vi "AlliGator Files Actions.vi"(0 "AlliGator Q Elements in":T7[](array[typedef]), 1 "VI in":refnum<vi>, 2 "Script in":bool, 5 "AlliGator IV DVR":refnum<data-value>, 7 "AlliGator Q Event in":T8=enum."GUI:Idle", 9 "Data":variant, 11 "error in (no error)":errorcluster, 12 "AlliGator Ctrl Refnums":T9) -> (3 "Script out":bool, 4 "AlliGator Q Elements out":T7[](array[typedef]), 6 "AlliGator IV DVR":refnum<data-value>, 10 "[Notebook Message]":T2[](array[typedef]) {"Message Style"."Font Size" min=6.0 step=1.0}, 15 "error out":errorcluster)   [LabVIEW 2021, in "AlliGator Action Engine.lvlib"]
doc: "Processes AlliGator files-related actions."
uses:
  AlliGator Action Engine.lvlib
  AlliGator Q Event.ctl
  GUI/AlliGator Ctrl Refnums.ctl
  GUI/AlliGator Other Ctrl Refnums.ctl
  GUI/AlliGator State Indicator.ctl
  GUI/AlliGator Main Window Tabs.ctl
  GUI/AlliGator Phasor Plot Ctrl Refnums.ctl
  GUI/AlliGator Phasor Graph Ctrl Refnums.ctl
  Phasor/Phasor Calibration Type.ctl
  GUI/AlliGator Dataset Ctrl Refnums.ctl
  Source Image/AlliGator Displayed Image.ctl
  GUI/AlliGator Registered Events Ctrl Refnums.ctl
  GUI/AlliGator Image Histogram Control Refnums.ctl
  Histograms/Linear Histogram Options.ctl
  Histograms/Histogram Bin Option.ctl
  Histograms/Histogram Bin Position.ctl
  Decay Fit Parameter Map/AlliGator Decay Fit Map Control Refnums.ctl
  Fits/IRF(X)PSED/Decay Fit Parameters & Derived Quantities List v2.ctl
  Parameter Map/AlliGator Parameter Map Control Refnums.ctl
  AlliGator Q Element.ctl
  Internal Variables/AlliGator Internal Variables v2.ctl
  <vilib>/vision/Image Controls.llb/IMAQ Image.ctl
  Internal Variables/AlliGator Gate Image Set.ctl
  Files/AlliGator FLI Dataset Type.ctl
  Files/AlliGator Data Series Type.ctl
  Dual-Channel Datasets/AlliGator Dataset Channel.ctl
  Settings/AlliGator Gate Arithmetic.ctl
  Image/Named ROI Description.ctl
  Phasor Graph/AlliGator Decay Metadata v3.ctl
  Decay Analysis/Decay Preprocessing/AlliGator Decay Background Subtraction Info.ctl
  Decay Analysis/Decay Preprocessing/AlliGator Baseline Subtraction Method.ctl
  Graphs/XY Graph/XY Graph Plot Shift Parameters.ctl
  Graphs/XY Graph/XY Graph Plot Shift Method.ctl
  Decay Analysis/Decay Preprocessing/AlliGator Decay Extrapolation Parameters.ctl
  Phasor/Calibration Phasor (m, phi).ctl
  Phasor/Phasor Reference Series.ctl
  Phasor/Phasor Calibration Map v2.ctl
  Phasor/Phasor (g, s).ctl
  Phasor Graph/AlliGator Raw Phasor Plot Data v5.ctl
  Phasor/Phasor Standard Deviation Options.ctl
  Phasor Plot/AlliGator Phasor Multi-Harmonic Data.ctl
  Phasor/Phasor Harmonic Data.ctl
  Decay Fit Parameter Map/AlliGator Decay Fit Options & Parameters v4.ctl
  Fits/IRF(X)PSED/Decay Fit Options v4.ctl
  Fits/Decay Convolution/Decay Model.ctl
  Fits/Residual Type.ctl
  Fits/IRF(X)PSED/Fit Weights Type v2.ctl
  Fits/Non-linear Fitting Method v2.ctl
  Fits/Fit Calculation Method.ctl
  Fits/Non-linear Fitting Algorithm.ctl
  Decay Analysis/Decay Fit/AlliGator Decay Fit Parameter Constraints 2.ctl
  Fits/IRF(X)PSED/Decay Fit Parameters In List.ctl
  Fits/IRF(X)PSED/MLE Baseline Offset Type.ctl
  Decay Analysis/Decay Preprocessing/AlliGator Decay Preprocessing Parameters.ctl
  Fits/IRF(X)PSED/Decay Fit Result Constraint.ctl
  Decay Fit Parameter Map/AlliGator Parameter Maps Data.ctl
  Notebook/Notebook Message Object.ctl
  Rich Text Box/Text Formatting.ctl
  Rich Text Box/Text Colors.ctl
  Rich Text Box/Text Style.ctl
  Rich Text Box/Text Alignment.ctl
  Rich Text Box/Text Format List.ctl
  GUI/AlliGator Windows List.ctl
  Alligator Elements Order in Action Stack.ctl
  Files/AlliGator Export Dataset Options.ctl
  Globals, Variables, Constants/AlliGator Variables List.ctl
  Files/AlliGator Load Dataset Options.ctl
  Files/AlliGator Single Image File Info.ctl
  Source Image/AlliGator Image Type.ctl
  Files/AlliGator Folder Selection.ctl
  Files/AlliGator Select Folder Mode.ctl
  Scripts/AlliGator Data Load & Process Options.ctl
  Scripts/AlliGator Data Information.ctl
  Settings/AlliGator Background Subtraction Parameters.ctl
  Settings/AlliGator Define Gates to.ctl
  Settings/AlliGator Gates to Keep.ctl
  Scripts/AlliGator Source Image Settings.ctl
  Settings/AlliGator Low Count Pixels Rejection Options.ctl
  Settings/AlliGator High Count Pixels Rejection Options.ctl
  Settings/AlliGator Image Smoothing Options.ctl
  Arrays/Kernel Type.ctl
  Arrays/Smoothing Algorithm.ctl
  Source Image/AlliGator Image Binning Options.ctl
  Decay Analysis/Decay Preprocessing/AlliGator Decay Preprocessing Options.ctl
  Decay Analysis/Decay Preprocessing/AlliGator Background Subtraction Parameters.ctl
  Settings/AlliGator Settings List.ctl
  Globals, Variables, Constants/AlliGator Globals.vi
  AlliGator Add Action Array to Stack.vi
  Variant/Variant to Data/Variant to I32.vi
  Variant/Variant to Data/Variant to Path.vi
  AlliGator Add Single Action to Stack.vi
  Variant/Variant to Data/Variant to DBL.vi
  Variant/Variant to Data/Variant to Data.lvlib
  GUI/AlliGator GUI.lvlib
  Utilities/Utilities.lvlib
  GUI/GUI.lvlib
  Files/AlliGator Files.lvlib
  Source Image/AlliGator Source Image.lvlib
  Scripts/AlliGator Scripts.lvlib
  Graphs/XY Graph/XY Graph Add-Ons.lvlib
  Decay Analysis/Decay Preprocessing/AlliGator Decay Preprocessing.lvlib
  Arrays/Arrays.lvlib
  Settings/AlliGator Settings.lvlib
  Globals, Variables, Constants/AlliGator Globals, Variables & Constants.lvlib
  Image/Image.lvlib
  Notebook/Notebook.lvlib
  Phasor/Phasor.lvlib
  Decay Fit Parameter Map/AlliGator Decay Fit Parameter Map.lvlib
  Phasor Graph/AlliGator Phasor Graph.lvlib
  Internal Variables/AlliGator Internal Variables.lvlib
  Phasor Plot/AlliGator Phasor Plot.lvlib
  Fits/Fits.lvlib
  Decay Analysis/Decay Fit/AlliGator Decay Fit.lvlib
  Rich Text Box/Rich Text Box.lvlib
  Dual-Channel Datasets/AlliGator Dual-Channel Datasets.lvlib
  Histograms/Histogram Window.lvlib
  Parameter Map/AlliGator Parameter Map.lvlib
panel:
  in  "Displayed Image 2":T1=enum."Sum of All Gates" caption="Displayed Image"
  in  "Displayed Image":T1=enum."Sum of All Gates"
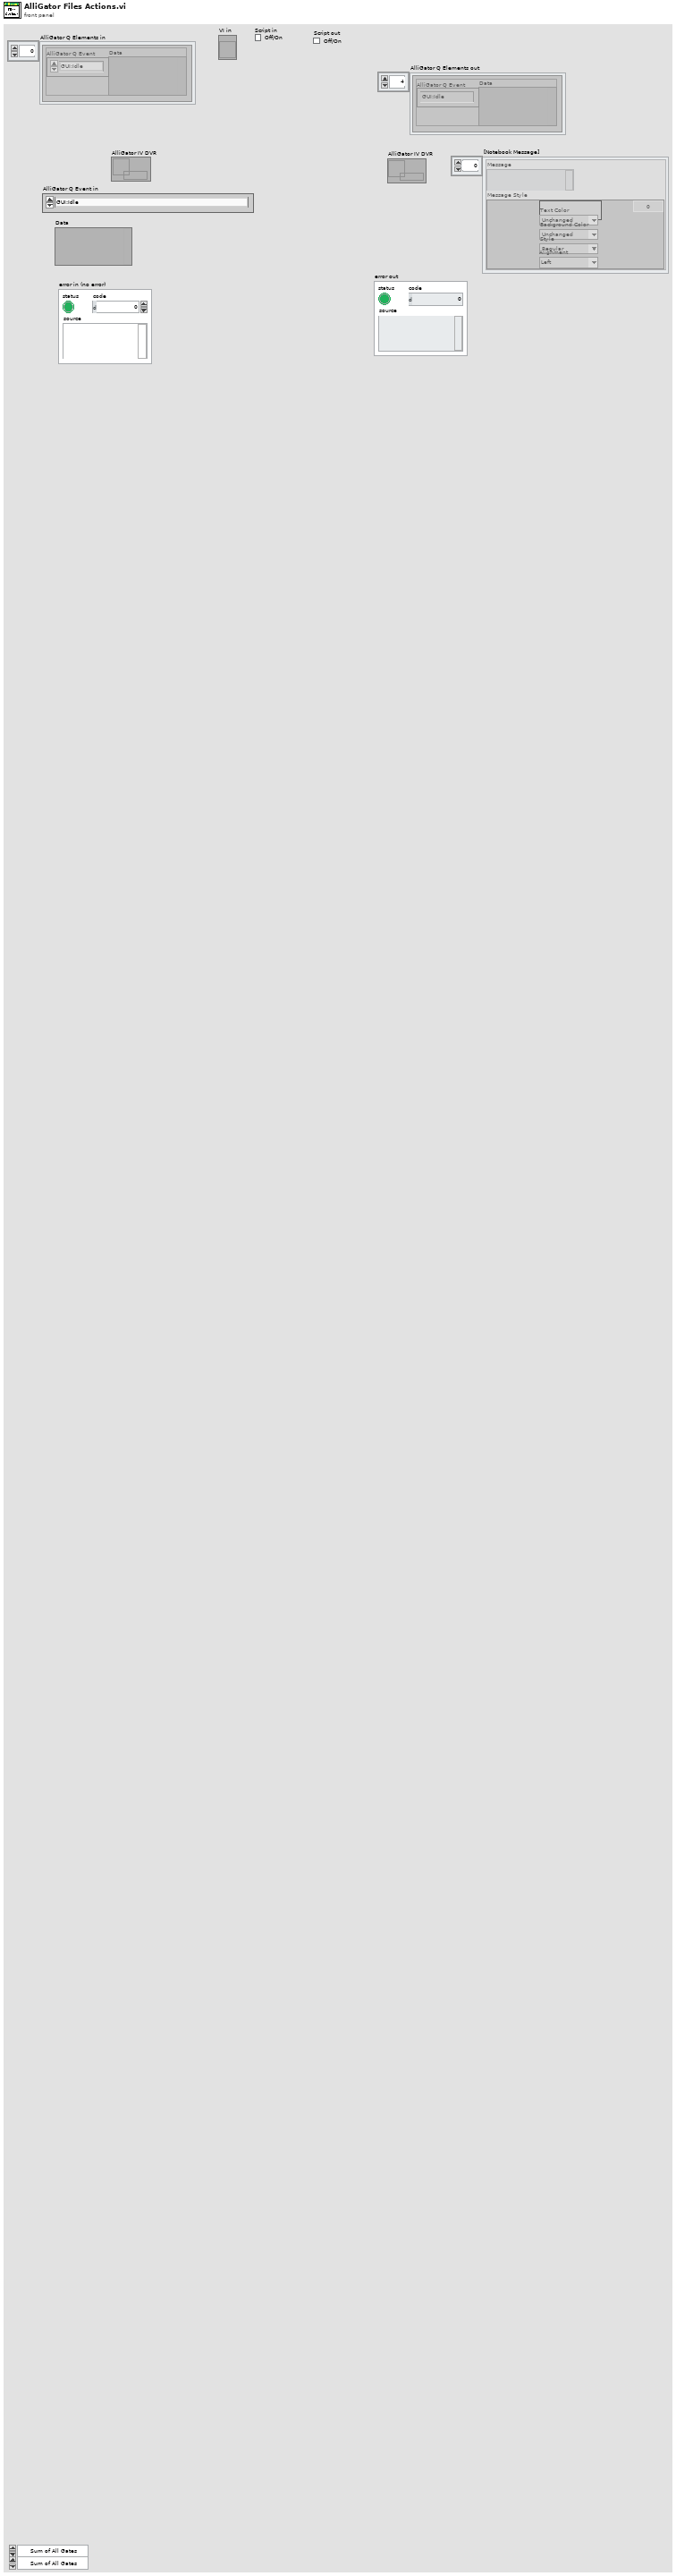
[diagram p1: front panel]
types:
  T1 = typedef "AlliGator Source Image.lvlib/AlliGator Displayed Image.ctl" = enum16{"Single Gate", "Sum of All Gates", "Max of All Gates", "Min of All Gates", "-", "White Ligth Image", "Mask Image"}
  T2 = typedef "Notebook.lvlib/Notebook Message Object.ctl" = cluster{"Message":string, "Message Style":T3}
  T3 = typedef "Rich Text Box.lvlib/Text Formatting.ctl" = cluster{"Font":string, "Text Color":T4, "Background Color":T4, "Style":T5, "Font Size":dbl, "Alignment":T6}
  T4 = typedef "Rich Text Box.lvlib/Text Colors.ctl" = enum16{"Unchanged", "Black", "Blue", "Cyan", "Maroon", "Gray", "Violet", "Green", "Light Green", "Orange", "Yellow", "Magenta", "Red", "White"}
  T5 = typedef "Rich Text Box.lvlib/Text Style.ctl" = enum16{"Regular", "Bold", "Italic", "Underline", "Strikeout"}
  T6 = typedef "Rich Text Box.lvlib/Text Alignment.ctl" = enum16{"Left", "Right", "Center"}
  T7 = typedef "AlliGator Action Engine.lvlib/AlliGator Q Element.ctl" = cluster{"AlliGator Q Event":T8, "Data":variant}
  T8 = typedef "AlliGator Action Engine.lvlib/AlliGator Q Event.ctl" = enum16{"---- Files ----", "Files:Set Batch Export Files To Save", "Files:Set Dataset Loading & Pre-processing Options", "Files:Check #Frames in Dataset", "Files:Increment Frame Index", "Files:Open Mask Image", "Files:Open White Light Image", "Files:Open Single Dataset", "Files:New Folder of Folders Selected", "Files:Load File (all Types)_Scriptable", "Files:Move Flattened Series to Folders Series", "Files:Select Folder", "Files:Load FLI Dataset", "Files:Load Swiss SPAD 1 Dataset", "Files:Load Swiss SPAD 2 Dataset", "Files:Load .sdt FLI Dataset", "Files:Load .ptu FLI Dataset", "Files:Load .bin FLI Dataset", "Files:Load Single Gate Image Folder", "Files:Load I/m/phi Dataset (deprecated)", "Files:Load Single Image", "Files:Subtract Background File", "Files:Export FLI Dataset", "Files:Load HDF5 FLI Dataset", "Files:Set Destination File Path", "Files:Save Mask Image", "Files:Batch Conversion", "Files:New Folder Selected", "Files:Close FLI Dataset", "Files:Close FLI Dataset Series", "Files:Close White Light Image", "Files:Close Mask Image", "---- FLI Dataset ----", "FLI Dataset:Channel Arithmetic", "FLI Dataset:Export Average Lifetime Map as ASCII", "FLI Dataset:Export User-Defined Quantity Map as ASCII", "FLI Dataset:Python Function FLI Dataset Event", "FLI Dataset:ROI Analysis", "FLI Dataset:Tilted Logistic Square Gated IRF Characteristics Map", "FLI Dataset:Logistic Square Gated IRF Characteristics Map", "FLI Dataset:Square Gated IRF Characteristics Map", "FLI Dataset:Multi-ROI Single-Pixel Phasor Analysis", "FLI Dataset:Multi-ROI Single-Pixel NLSF Analysis", "FLI Dataset:All ROIs IRF Extraction", "FLI Dataset:All ROIs Decay Fit Non-Interactive (Fast + Individual IRF)", "FLI Dataset:All ROIs Phasor Analysis", "FLI Dataset:All ROIs Decay Fit", "FLI Dataset:Fluorescence Decay Statistics", "FLI Dataset:Update Decay Statistics Graph", "FLI Dataset:Get Decay from ROI", "FLI Dataset:All ROIs Average Lifetimes", "FLI Dataset:Save/Load Local IRFs", "FLI Dataset:Clear Local IRFs", "FLI Dataset:Phasor Calibration Maps (# Gates Series) Script", "FLI Dataset:Calibrated Phasor Map Series", "---- FLI Dataset Series ----", "FLI Dataset Series:Sum All Datasets in Series", "FLI Dataset Series:Add Dataset to Accumulated Dataset", "FLI Dataset Series:Display Accumulated Dataset", "FLI Dataset Series:Clear Dataset Series Sum", "FLI Dataset Series:Time-Series Analysis (NLSF)", "FLI Dataset Series:Time-Series Analysis (Phasor)", "---- Image ----", "Image:Update Image Profile Plots", "Image:Image Histogram Cursor Move", "Image:Image Histogram", "Image:Image Contrast", "Image:Set Image Histogram Cursor Move Flag", "Image:Clear Image Overlay", "Image:Use ROI as Search Area", "Image:Set ROI Diameter", "Image:Save Image Data as TIFF", "Image:Save Displayed Image with Overlay", "Image:Save Image Overlay Only", "Image:Save Image as Hot Pixel Mask", "Image:Change Source Image Color Palette", "Image:Copy Image to Clipboard", "Image:Source Image ROI Selection", "Image:Delete All ROIs", "Image:Delete All Unselected ROIs", "Image:Delete ROI", "Image:Merge All ROIs", "Image:Store ROI", "Image:Source Image ROI Storage", "Image:Export ROI Description to Notebook", "Image:Save ROI", "Image:Load ROI", "Image:Paste ROI Definition", "Image:Clear ROI", "Image:Identify ROIs in Mask Image", "Image:Create Complementary ROI", "Image:Create Contour ROI", "Image:Create ROI(s) from Pixels with Peak above Min_Scriptable", "Image:Create ROI(s) from Pixels with Intensity above Min_Scriptable", "Image:Compute ROI Statistics", "Image:Delete ROI(s) based on ROI Characteristics", "Image:Create ROI Grid", "Image:ROI to Individual Pixel ROIs", "Image:Python Function Source Image Event", "Image:Show Phasor Calibration Map ROI Centers", "Image:Convert ROI to Mask Image", "Image:Mouse Move", "Image:Mouse Up", "Image:Set Source Image Mouse Move Flag", "Image:Add Scale Bar Overlay", "Image:Delete Existing ROIs Option", "Image:Overlay ROI Median", "Image:Check Current ROI", "Image:Update True Pixel Value", "---- Decay ----", "Decay:Clear IRF/Reference Plot", "Decay:Add Decay to Graph", "Decay:Smoothen Plot", "Decay:Smoothen Plot Tail", "Decay:Average Selected Plots", "Decay:Extract IRF", "Decay:Optimal IRF Extraction", "Decay:Threshold IRF", "Decay:Fit to Model IRF", "Decay:Fit IRF to Square Gate", "Decay:Fit IRF to Logistic Square Gate", "Decay:Fit IRF to Tilted Logistic Square Gate", "Decay:Create Bounding Cursors Set", "Decay:Export Bounding Cursors Definition to Notebook", "Decay:Denoise Plot", "Decay:Compute Cumulative Function", "Decay:Use as Reference Decay", "Decay:Show Reference Decay/IRF", "Decay:Extrapolate Decay", "Decay:Create Head & Tail Bounding Cursors", "Decay:Store Cursor-defined Head & Tail Fractions", "Decay:Rebin Plot", "Decay:1-Normalize Decay", "Decay:[0-1]-Normalize Plot", "Decay:Straighten Decay", "Decay:Shift Decay", "Decay:Fold Decay", "Decay:Fit Decay", "Decay:Global Fit of Selected Decays", "Decay:Post Global Fit Script", "Decay:Add Global Fit Parameters to Graph", "Decay:Add Decay Parameter(s) to Plot (Graph)", "Decay:Export Decay to Phasor Graph", "Decay:Compute Average Lifetime", "Decay:Plot Convolution", "Decay:Graph Tip Strip Update", "---- Decay Statistics ----", "Decay Statistics:Tip Strip Update", "---- Intensity Time Trace ----", "Intensity Time Trace:Use File Timestamp", "Intensity Time Trace:Load Intensity Corrections File", "Intensity Time Trace:Clear Intensity Corrections File", "Intensity Time Trace:Tip Strip Update", "---- Phasor Plot ----", "Phasor Plot:Build Phasor Plot", "Phasor Plot:Change Phasor Plot Color Palette", "Phasor Plot:Adjust Phasor Plot Display Range", "Phasor Plot:Highlight Image ROI in Phasor Plot", "Phasor Plot:Save Phasor Plot Image with Overlay", "Phasor Plot:Export Complex Phasor Map", "Phasor Plot:Export Phasor Ratio Map", "Phasor Plot:Export Average Lifetime Map", "Phasor Plot:Compute Phase Lifetime Histogram", "Phasor Plot:Compute Phasor Ratio Histogram", "Phasor Plot:Compute Phase Lifetime vs Intensity Scatter Plot", "Phasor Plot:Weber 2-Component Decomposition", "Phasor Plot:Update Phasor Color Map Vertices", "Phasor Plot:Clear Phasor Overlay", "Phasor Plot:Use Segment Extremities as References", "Phasor Plot:Use UC/Segment Intersections as References", "Phasor Plot:Use UC/Principal Axis Intersections as References", "Phasor Plot:Use UC/Linear Fit Intersections as References", "Phasor Plot:Update Phasor Plot Reference", "Phasor Plot:Show Local Phasor Info in Phasor Plot", "Phasor Plot:Update Phasor Plot State", "Phasor Plot:Phasor Plot ROI Storage", "Phasor Plot:Phasor Plot ROI Selection", "Phasor Plot:Python Function Phasor Plot Event", "Phasor Plot:Overlay Phasor ROI, Ratio or Map in Source Image", "Phasor Plot:Compute Decay of Selected Phasors", "Phasor Plot:Phasor at Image Pixel", "Phasor Plot:Mouse Move", "Phasor Plot:Mouse Up", "Phasor Plot:Display Range Mouse Move", "Phasor Plot:Set Mouse Move Flag", "Phasor Plot:Update True Phasor Plot Value", "---- Phasor Graph ----", "Phasor Graph:Get Phasor Value", "Phasor Graph:Create New Phasor Plot Dialog", "Phasor Graph:Update Last Phasor Value", "Phasor Graph:Update Phasor (m, phi)", "Phasor Graph:Remove Single Phasor from Plot", "Phasor Graph:Add Single Phasor to Plot", "Phasor Graph:Remove Phasor Plot", "Phasor Graph:Remove Selected Phasor Plots", "Phasor Graph:Clear Phasor Data", "Phasor Graph:Clear Phasor Graph", "Phasor Graph:Cursor Move", "Phasor Graph:Draw Cursor Connecting Line", "Phasor Graph:Clear Cursor Connecting Line", "Phasor Graph:Find UC Intersection", "Phasor Graph:Use UC/Cursor-Defined Line Intersections", "Phasor Graph:Use Selected Plots Fitted Line/UC Intersections", "Phasor Graph:Use Selected Plots Principal Axis/UC Intersections", "Phasor Graph:Show Single Phasor", "Phasor Graph:Save Single Phasor Plot", "Phasor Graph:Save All Phasor Plots", "Phasor Graph:Load Phasor Plot(s)", "Phasor Graph:Phasor Multiplication", "Phasor Graph:Compute Average Phasor", "Phasor Graph:Compute Multiple Average Phasors (Selected Plots)", "Phasor Graph:Export Single Phasor Plot Phase Lifetimes", "Phasor Graph:Parameter 2 vs Parameter 1 Scatter Plot", "Phasor Graph:Use Cursor n Location", "Phasor Graph:Set Reference n to Current Phase Lifetime Value", "Phasor Graph:Set Reference n to Lifetime Value", "Phasor Graph:Set Cursor n Location", "Phasor Graph:Save Phasor Graph Image", "Phasor Graph:Update SEPL Plot", "Phasor Graph:Export Single Phasor Plot Data", "Phasor Graph:Export Selected Phasor Plots Data", "Phasor Graph:Python Function Phasor Graph Event", "Phasor Graph:Tip Strip Update", "---- Calibration ----", "Calibration:Set Calibration Type", "Calibration:Load/Save Phasor Calibration", "Calibration:Load/Save Phasor Calibration Series", "Calibration:Load/Save Phasor Calibration Map", "Calibration:Use as Calibration", "Calibration:Compute Optimal Calibration from Phasor References", "Calibration:Clear Phasor Calibration", "Calibration:Single Phasor Calibration Information", "Calibration:Use as Calibration Series", "Calibration:Use as Calibration Map", "Calibration:Clear Calibration Series", "Calibration:Phasor Calibration Series Information", "Calibration:Clear Calibration Map", "Calibration:Phasor Calibration Map Information", "Calibration:Apply Phasor Calibration", "Calibration:Update Single Plot Calibration", "Calibration:Update Multiple Plots Calibration", "Calibration:Clear Single Plot Calibration", "Calibration:Clear All Plots Calibrations", "Calibration:Clear Plot(s) Calibration(s)?", "---- Phasor Ratio ----", "Phasor Ratio:Clear Reference n", "Phasor Ratio:Toggle Selected Plot(s)  Lock to Reference 1", "Phasor Ratio:Use as Reference n", "Phasor Ratio:Send Reference n to Notebook", "Phasor Ratio:Toggle Selected Plot(s)  Lock to Reference 2", "Phasor Ratio:Compute Phasor Ratio at Mouse Location", "Phasor Ratio:Compute Phasor Plot's Average Phasor Ratio", "Phasor Ratio:Compute Time-Series Phasor Ratios", "Phasor Ratio:Fit Line to Phasor Ratio Plot", "Phasor Ratio:Save References", "Phasor Ratio:Load References", "Phasor Ratio:Update Phasor Reference 1", "Phasor Ratio:Update Phasor Reference 2", "Phasor Ratio:Move Cursor n to Reference n", "Phasor Ratio:Use as Phasor Reference 1 Lifetime", "Phasor Ratio:Use as Phasor Reference 2 Lifetime", "Phasor Ratio:Export Phasor Ratio Map as ASCII", "Phasor Ratio:Tip Strip Update", "---- Lifetime & Other Parameters Graph ----", "Lifetime:Compute Sliced Mean, SDV and CV Plots", "Lifetime:Plot Decay Shifts", "Lifetime:Plot Histogram", "---- Decay Fit Parameter Map ----", "Decay Fit Parameter Map:Export ROI NLSF Data as ASCII", "Decay Fit Parameter Map:Set Decay Fit Parameter Map Selection", "Decay Fit Parameter Map:Build Decay Fit Parameter Map", "Decay Fit Parameter Map:Change Decay Fit Parameter Map Color Palette", "Decay Fit Parameter Map:Export Decay Fit Parameter Map Data as ASCII", "Decay Fit Parameter Map:Export All Decay Fit Parameter Maps Data as ASCII", "Decay Fit Parameter Map:Selected Parameter Scatterplot", "Decay Fit Parameter Map:Parameter 2 vs Parameter 1 Scatterplot", "Decay Fit Parameter Map:Save Decay Fit Parameter Map Image", "Decay Fit Parameter Map:Save-Load IRFs & Fit Data", "Decay Fit Parameter Map:Update Local Decay Plots", "Decay Fit Parameter Map:Python Function Decay Fit Parameters Map Event", "Decay Fit Parameter Map:Overlay Decay Fit Parameter Map in Source Image", "Decay Fit Parameter Map:Selected Parameter vs Intensity Scatterplot", "Decay Fit Parameter Map:Mouse Up", "Decay Fit Parameter Map:Mouse Move", "Decay Fit Parameter Map:Display Range Mouse Move", "Decay Fit Parameter Map:Change Map Resolution", "Decay Fit Parameter Map:Variance Significance Maps", "Decay Fit Parameter Map:Fit Result Constraints Window", "---- Parameter Map ----", "Parameter Map:Export ROI Parameters Data as ASCII", "Parameter Map:Add Parameter Map Set", "Parameter Map:Delete Parameter Map Set", "Parameter Map:Update Parameter List", "Parameter Map:Build Parameter Map", "Parameter Map:Change Parameter Map Color Palette", "Parameter Map:Export Parameter Map Data as ASCII", "Parameter Map:Export All Parameter Maps Data as ASCII", "Parameter Map:Selected Parameter Scatterplot", "Parameter Map:Parameter 2 vs Parameter 1 Scatterplot", "Parameter Map:Selected Parameter vs Intensity Scatterplot", "Parameter Map:Save Parameter Map Image", "Parameter Map:Save-Load IRFs & Parameter Maps (TODO)", "Parameter Map:Set Parameter Map Selection", "Parameter Map:Python Function Parameter Map Event", "Parameter Map:Overlay Parameter Map in Source Image", "Parameter Map:Update Local Decay Plots", "Parameter Map:Mouse Up", "Parameter Map:Mouse Move", "Parameter Map:Display Range Mouse Move", "---- Generic Graph ----", "Generic Graph:Generic XY Graph Event", "Generic Graph:Python Function XY Graph Event", "Generic Graph:New Plot", "Generic Graph:Save Plot", "Generic Graph:XY Plot Histogram", "Generic Graph:Set XY Graph Plot Name", "Generic Graph:Set Last Cursor Style", "Generic Graph:Tip Strip Update", "---- GUI ----", "GUI:Start Script", "GUI:Type of Displayed Image Changed", "GUI:Gate Image Slide Changed", "GUI:Show Busy Icon", "GUI:Show Busy Icon & Abort Button", "GUI:Hide Busy Icon", "GUI:Hide Busy Icon & Abort Button", "GUI:Abort", "GUI:End Script", "GUI:Start Timing", "GUI:End Timing", "GUI:Set State Indicator", "GUI:Send Parameters JSON Strings to Clipboard", "GUI:Set Gate Step", "GUI:Idle", "GUI:Initialization", "GUI:Quit", "GUI:Increment Dataset Index", "GUI:Set Dataset Index to -1", "GUI:Time Series Slider Moved", "GUI:Time Series Slider Changed", "GUI:Toggle Playback or Loop", "GUI:Playback Script", "GUI:Set Phasor Frequency", "GUI:Open Window", "GUI:Start Test Script", "GUI:End Test Script", "GUI:Set Verbose Mode", "GUI:Set Verbose Settings Mode", "DEBUG"}
  T9 = typedef "AlliGator GUI.lvlib/AlliGator Ctrl Refnums.ctl" = cluster{"Other AlliGator Ctrl Refnums":T10, "Phasor Plot Ctrl Refnums":T11, "Phasor Graph Ctrl Refnums":T12, "Dataset Control Refnums":T13, "Registered Events Ctrl Refnums":T14, "Image Histogram Ctrl Refnums":T15, "Decay Fit Map Ctrl Refnums":T16, "Parameter Map Ctrl Refnums":T17}
  T10 = typedef "AlliGator GUI.lvlib/AlliGator Other Ctrl Refnums.ctl" = cluster{"State Indicators":refnum<vi>, " Progress Bar":refnum<vi>, "Decay Graph Active":refnum<vi>, "Decay Statistics Bin":refnum<vi>, "Time Step":refnum<vi>, "Use File Timestamp":refnum<vi>, "Tab Control":refnum<vi>, "CPU":refnum<vi>, "Abort Fit":refnum<vi>, "Dataset File/Folder Path":refnum<vi>, "Abort ROI Creation":refnum<vi>, "Event LED":refnum<vi>, "Dataset File/Folder Path 2":refnum<vi>, "Dataset File/Folder Path 3":refnum<vi>, "Dataset File/Folder Path 4":refnum<vi>, "Dataset File/Folder Path 5":refnum<vi>, "Dataset File/Folder Path 6":refnum<vi>, "Dataset File/Folder Path 7":refnum<vi>, "Dataset File/Folder Path 8":refnum<vi>, "Dataset File/Folder Path 9":refnum<vi>, "Dataset File/Folder Path 10":refnum<vi>, "Dataset File/Folder Path 11":refnum<vi>}
  T11 = typedef "AlliGator GUI.lvlib/AlliGator Phasor Plot Ctrl Refnums.ctl" = cluster{"Phasor Ratio":refnum<vi>, "Modulus Lifetime":refnum<vi>, "Phasor at cursor (m, phi)":refnum<vi>, "Phase Lifetime":refnum<vi>, "Phasor at cursor (g, s)":refnum<vi>, "Phasor Plor Average Lifetime":refnum<vi>, "Phasor Plot Active":refnum<vi>, "Save Phasor Plot":refnum<vi>, "Image Overlay Color":refnum<vi>, "Phasor Plot Color Scale":refnum<vi>, "Reference 1 Button":refnum<vi>, "Reference 2 Button":refnum<vi>, "True Phasor Plot Value":refnum<vi>}
  T12 = typedef "AlliGator GUI.lvlib/AlliGator Phasor Graph Ctrl Refnums.ctl" = cluster{"Phasor Ratio":refnum<vi>, "Modulus Lifetime":refnum<vi>, "Phasor at cursor (m, phi)":refnum<vi>, "Phase Lifetime":refnum<vi>, "Phasor at cursor (g, s)":refnum<vi>, "Phasor Graph Average Lifetime":refnum<vi>, "Phasor Graph Active":refnum<vi>, "Save Phasor Graph":refnum<vi>, "Phasor Frame Slide":refnum<vi>, "Single Step Phasor":refnum<vi>, "Calibration Type":refnum<vi>, "Show Line":refnum<vi>, "Phase Lifetime 1":refnum<vi>, "Phase Lifetime 2":refnum<vi>, "Phasor Graph Frequency":refnum<vi>, "Phasor Reference 1 Control":refnum<vi>, "Phasor Reference 2 Control":refnum<vi>, "Calibration Lifetime":refnum<vi>, "Phase Lifetime SDV":refnum<vi>, "Average Lifetime SDV":refnum<vi>, "Phasor Ratio SDV":refnum<vi>, "Modulus Lifetime SDV":refnum<vi>}
  T13 = typedef "AlliGator GUI.lvlib/AlliGator Dataset Ctrl Refnums.ctl" = cluster{"Current Data":refnum<vi>, "Gate Image Slide":refnum<vi>, "Time Point Slide":refnum<vi>, "Current Time Stamp":refnum<vi>, "Save Image":refnum<vi>, "Displayed Image":refnum<vi>, "Overlay Mode":refnum<vi>, "Phasor Overlay Color":refnum<vi>, "Image Color Scale":refnum<vi>, "Use ROI as Search Area":refnum<vi>, "Source Image ROI Color":refnum<vi>, "True Pixel Value":refnum<vi>}
  T14 = typedef "AlliGator GUI.lvlib/AlliGator Registered Events Ctrl Refnums.ctl" = cluster{"Time Point Slider":refnum<vi>, "Phasor Plot Display Range":refnum<vi>, "Decay Graph":refnum<vi>, "Decay Statistics Graph":refnum<vi>, "Intensity Time Trace":refnum<vi>, "Phasor Graph":refnum<vi>, "Phasor Ratio Graph":refnum<vi>, "Lifetime Graph":refnum<vi>, "Phasor Plot Display":refnum<vi>, "Source Image Display":refnum<vi>, "Decay Fit Parameter Map Display Range":refnum<vi>, "Decay Fit Parameter Map Display":refnum<vi>, "Parameter Map Display Range":refnum<vi>, "Parameter Map Display":refnum<vi>, "Phasor Plot Display Range":refnum<vi>}
  T15 = typedef "AlliGator GUI.lvlib/AlliGator Image Histogram Control Refnums.ctl" = cluster{"Image Histogram":refnum<vi>, "Image Histogram Options":refnum<vi>, "Image Histogram Active":refnum<vi>, "Image Histogram Upper Percentile":refnum<vi>, "Image Histogram Lower Percentile":refnum<vi>, "Auto-Adjust Contrast":refnum<vi>}
  T16 = typedef "AlliGator Decay Fit Parameter Map.lvlib/AlliGator Decay Fit Map Control Refnums.ctl" = cluster{"Decay Fit Parameter Map Color Scale":refnum<vi>, "Decay Fit Parameter":refnum<vi>, "Max Parameter":refnum<vi>, "Min Parameter":refnum<vi>, "Decay Fit Parameter Map Display":refnum<vi>, "Decay Fit Parameter Map Display Range":refnum<vi>, "Decay Parameter Map X":refnum<vi>, "Decay Parameter Map Y":refnum<vi>, "Decay Parameter Map Value":refnum<vi>}
  T17 = typedef "AlliGator Parameter Map.lvlib/AlliGator Parameter Map Control Refnums.ctl" = cluster{"Parameter Map Color Scale":refnum<vi>, "Map Parameter":refnum<vi>, "Max Parameter":refnum<vi>, "Min Parameter":refnum<vi>, "Parameter Map Display":refnum<vi>, "Parameter Map Display Range":refnum<vi>, "Parameter Map Set":refnum<vi>, "Parameter Map X":refnum<vi>, "Parameter Map Y":refnum<vi>, "Parameter Map Value":refnum<vi>}
  T18 = typedef "Notebook.lvlib/Text Format List.ctl" = enum16{"Message", "Result", "Error", "Setting", "Verbose", "Warning"}
  T19 = typedef "AlliGator GUI.lvlib/AlliGator Windows List.ctl" = enum16{"AlliGator Window", "Settings Window", "Notebook Window", "Dataset Information Window", "Source Image ROI Manager Window", "Phasor Plot ROI Manager Window", "Phasor Harmonic Manager Window", "Histogram Window", "Image Profile Window", "Local Decay Window", "About Window", "Batch Conversion Window", "Shot Noise Influence on Average Lifetime", "Fit Method Benchmark", "Camera Noise Influence on Lifetime", "AlliGator Alias Definition", "Fit Result Constraints Window"}
  T20 = typedef "AlliGator Action Engine.lvlib/Alligator Elements Order in Action Stack.ctl" = enum16{"Enqueue 2 AFTER 1", "Enqueue 2 BEFORE 1"}
  T21 = typedef "AlliGator Files.lvlib/AlliGator Export Dataset Options.ctl" = cluster{"Destination File Type":string, "Dialog?":bool}
  T22 = typedef "AlliGator Files.lvlib/AlliGator Load Dataset Options.ctl" = cluster{"FLI Dataset Type":T23, "No Dialog?":bool, "File Path":path}
  T23 = typedef "AlliGator Files.lvlib/AlliGator FLI Dataset Type.ctl" = enum16{"HDF5 FLI Dataset", "Gate Image Folder", ".sdt FLI Dataset (Becker & Hickl)", ".ptu FLI Dataset (PicoQuant)", "SS1 FLI Dataset", "SS2 FLI Dataset", "I/m/phi Dataset", ".bin FLI Dataset (PicoQuant Binned)", ".bin FLI Dataset (Piccolo Binned)", ".mat FLI Dataset"}
  T24 = typedef "AlliGator Files.lvlib/AlliGator Single Image File Info.ctl" = cluster{"Image Type":T25, "Image Path":path}
  T25 = typedef "AlliGator Source Image.lvlib/AlliGator Image Type.ctl" = enum16{"White Light Image", "Mask Image"}
  T26 = typedef "AlliGator Files.lvlib/AlliGator Folder Selection.ctl" = cluster{"Folder Selection Mode":T27, "Folder Path":path}
  T27 = typedef "AlliGator Files.lvlib/AlliGator Select Folder Mode.ctl" = enum16{"Select Gate Folder", "Select Folder of Gate Folders", "Select Folder of SwissSPAD 2 Datasets", "Select Folder of .sdt FLI Datasets (Becker & Hickl)", "Select Folder of .ptu FLI Datasets (PicoQuant)", "Select Folder of .bin FLI Datasets (PicoQuant Binned)", "Select Folder of .bin FLI Datasets (Piccolo Binned)", "Select Folder of HDF5 FLI Datasets"}
  T28 = typedef "AlliGator Scripts.lvlib/AlliGator Data Load & Process Options.ctl" = cluster{"Data Information":T29, "Source Image Settings":T34, "Decay Preprocessing Options & Parameters":T41, "Clear Phasor Graph":bool}
  T29 = typedef "AlliGator Scripts.lvlib/AlliGator Data Information.ctl" = cluster{"Gates to Skip":T30, "# Gates":u32, "Gate Step":u32, "Gate Duration":dbl[unit], "Gate Separation":dbl[unit], "Pile-up Correction":bool, "Pixel Well Capacity":u32, "Define Gates to":T31, "Gates to Keep":T32, "Laser Period":dbl[unit], "SYNC Period":dbl[unit], "Channel Name":u16, "Channel Arithmetic":T33, "Background File Subtraction":bool, "Background Scaling Factor":dbl, "Background File":path, "Background Pile-up Correction":bool, "Background Pixel Well Capacity":u32, "Dataset Scaling Factor":dbl}
  T30 = typedef "AlliGator Settings.lvlib/AlliGator Background Subtraction Parameters.ctl" = cluster{"Start":u32, "End":u32}
  T31 = typedef "AlliGator Settings.lvlib/AlliGator Define Gates to.ctl" = enum32{"Skip", "Keep"}
  T32 = typedef "AlliGator Settings.lvlib/AlliGator Gates to Keep.ctl" = cluster{"First":u32, "Last":u32}
  T33 = typedef "AlliGator Settings.lvlib/AlliGator Gate Arithmetic.ctl" = enum16{"None", "INT-G2", "G2/INT*<INT>", "(1 - G2/INT)*<INT>"}
  T34 = typedef "AlliGator Scripts.lvlib/AlliGator Source Image Settings.ctl" = cluster{"Low Count Pixels Rejection Options":T35, "High Count Pixels Rejection Options":T36, "Peak Threshold":dbl, "Intensity Threshold":dbl, "Image Smoothing Options":T37, "Image Binning Options":T40}
  T35 = typedef "AlliGator Settings.lvlib/AlliGator Low Count Pixels Rejection Options.ctl" = cluster{"Background Low Threshold Factor":dbl, "Fixed Low Background Threshold":dbl, "Reject Low Count Pixels":bool, "Low Percentile":dbl}
  T36 = typedef "AlliGator Settings.lvlib/AlliGator High Count Pixels Rejection Options.ctl" = cluster{"Background High Threshold Factor":dbl, "Fixed High Background Threshold":dbl, "Reject High Count Pixels":bool, "High Percentile":dbl}
  T37 = typedef "AlliGator Settings.lvlib/AlliGator Image Smoothing Options.ctl" = cluster{"Use Image Smoothing":bool, "Kernel Type":T38, "Bin":i32, "Algorithm":T39}
  T38 = typedef "Arrays.lvlib/Kernel Type.ctl" = enum16{"Uniform", "Bilinear", "Gaussian"}
  T39 = typedef "Arrays.lvlib/Smoothing Algorithm.ctl" = enum16{"Rapid", "Thorough"}
  T40 = typedef "AlliGator Source Image.lvlib/AlliGator Image Binning Options.ctl" = cluster{"Use Image Binning":bool, "X Bin":i32, "Y Bin":i32}
  T41 = typedef "AlliGator Decay Preprocessing.lvlib/AlliGator Decay Preprocessing Options.ctl" = cluster{"Background Subtraction Parameters":T42, "Decay Preprocessing Parameters":T44, "Preprocessing Steps Order":string[]}
  T42 = typedef "AlliGator Decay Preprocessing.lvlib/AlliGator Background Subtraction Parameters.ctl" = cluster{"Background Definition Range":cluster{"Min Gate":dbl[unit], "Max Gate":dbl[unit]}, "Baseline Subtraction Method":T43, "Background Subtraction?":bool, "Background File":path, "Background Constant":dbl, "Background Scaling Factor":dbl, "Background Pile-up Correction":bool, "Background Pixel Well Capacity":u32}
  T43 = typedef "AlliGator Decay Preprocessing.lvlib/AlliGator Baseline Subtraction Method.ctl" = enum16{"Mean", "Min", "Square Gated Single-Exponential", "File", "Constant"}
  T44 = typedef "AlliGator Decay Preprocessing.lvlib/AlliGator Decay Preprocessing Parameters.ctl" = cluster{"Background Subtraction":bool, "Straighten Decay":bool, "Reverse Gates":bool, "1-Normalized Decay":bool, "Smoothen Decay":bool, "Smoothing Parameter":dbl, "Shift Decay":bool, "Decay Shift Parameters":T45, "Extrapolate Decay":bool, "Additional Points":u32, "Head Fraction":dbl, "Pixel-Normalize Decay":bool, "Use Periodicity":bool, "Use Cursors":bool, "Tail Fraction":dbl, "Use Decay Pre-Processing":bool, "Fold Decay":bool, "# Folds":u32, "[0-1]-Normalized Decay":bool}
  T45 = typedef "XY Graph Add-Ons.lvlib/XY Graph Plot Shift Parameters.ctl" = cluster{"Type":T46, "Shift":dbl[unit], "Threshold":dbl, "Rotate":bool}
  T46 = typedef "XY Graph Add-Ons.lvlib/XY Graph Plot Shift Method.ctl" = enum16{"Default", "CFD", "Threshold", "Cross-Correlation"}
  T47 = typedef "AlliGator Globals, Variables & Constants.lvlib/AlliGator Variables List.ctl" = enum16{"---- GUI ----", "GUI:Initialization Status", "GUI:State Indicators Refnum", "GUI:Original AlliGator Menu Items", "GUI:Current Action Loop State", "GUI:Script in progress", "GUI:Playback", "GUI:Loop Playback", "GUI:Search ROI Used", "GUI:Search ROI", "Decay Graph Max Legend Size", "Intensity Graph Max Legend Size", "Decay Statistics Graph Max Legend Size", "Phasor Graph Max Legend Size", "Phasor Ratio Graph Max Legend Size", "Lifetime Graph Max Legend Size", "---- Files ----", "Files:Export Dataset Frames as Individual Files", "Files:Show Batch Export Help Balloons", "Files:Frames in Dataset", "Files:ptu File Frame Start Indices", "Files:Current Frame in Dataset", "Files:Current Frame Timestamp", "Files:Dataset Loaded", "Files:Dataset Metadata", "Files:Dataset Channel", "Files:Dataset Data Description", "Files:Background Dataset Metadata", "Files:Background Dataset Channel", "Files:Background Dataset Data Description", "Files:Background File Subtraction", "Files:Background File Path", "Files:Background File Pile-up Correction", "Files:Background File Pixel Well Capacity", "Files:Background File Scaling Factor", "Files:Current Dataset Load Settings", "Files:Dataset Path", "Files:ICCD-specific Information", "Files:Macrotime Gate Separation", "------ Python Plugins ------", "Python Plugins:Information", "Python Plugins:Python Session", "Python Plugins:Valid Python Session?", "---- Source Image ----", "Source Image:ROIs", "Source Image:Current ROI", "Source Image:ROI Event Refnum", "X_Source Image:Display Range", "X_Source Image:Palette Information", "X_Source Image:Type of Displayed Image", "X_Time Gate Slider", "Source Image:Palette List", "Source Image:Scale", "Source Image:ROI Overlay Color", "Source Image:Overlay to Erase", "Source Image:Is Displayed Image Accumulated", "Source Image:White Light Image Modified", "Source Image:Mask Image Modified", "---- Image Profile Window ----", "Image Profile:Window Event Refnum", "Image Profile:IntensityType", "Image Profile:Intensity Average Type", "Image Profile:Intensity-weighted SDV", "Image Profile:Box Profile Type", "Image Profile:Window Open", "Image Profile:Plotted Fit Parameter", "------ Phasor Graph -------", "Phasor Graph:Show Line", "---- Phasor Plot ---", "Phasor Plot:Parameters Changed", "Phasor Plot:FLI Dataset Modified since last Calculation", "Phasor Harmonics Data", "Selected Phasor Harmonics", "Phasor Harmonic Manager Event Refnum", "Phasor Plot:ROIs", "Phasor Plot:Current ROI", "Phasor Plot:ROI Event Refnum", "Phasor Plot:Image Reference Points", "Phasor Plot:Computed", "Phasor Plot:Palette Information", "Phasor Plot:Palette List", "Phasor Plot:Phasor Ratio Palette Information", "Phasor Plot:Phasor Ratio Palette List", "Phasor Plot:Image Scale", "Phasor Plot:Image Overlay to Erase", "Phasor Plot:Image Elements to Update", "Phasor Plot:Current Calculation Parameters", "Phasor Plot:Current Calibration Options", "Phasor Plot:Reset Cumulated Phasor Plot", "Phasor Plot:Reference 1", "Phasor Plot:Lifetime Reference 1", "Phasor Plot:Reference 1 Frequency", "Phasor Plot:Reference 2", "Phasor Plot:Lifetime Reference 2", "Phasor Plot:Reference 2 Frequency", "---- Decay Analysis ----", "Number of Selected Decays to Fit", "LS Fit Results", "LAR Fit Results", "BS Fit Results", "Last Decay Max - Min", "Best Fit Parameters", "Best Fit Parameter Names", "Actual Size X", "Actual Size Y", "Binning X", "Binning Y", "Actual # Gates", "Dataset Number", "Gates to...", "Gates Skipped", "Gates to keep", "Gate Step", "Gate Separation", "Reversed Gates", "Pile-up Correction", "Pixel Well Capacity", "Background Subtracted", "Background Subtraction Method", "Background Definition Range", "Background File (deprecated)", "Number of Dataset Accumulated", "Array of Accumulated Dataset Paths", "Do Averaged Datasets", "Destination File Path", "Process Plot Target", "Use 1/D as Phasor Frequency", "---- Decay Fit Parameter Map -----", "Decay Fit Parameter Map:Palette Information", "Decay Fit Parameter Map:Palette List", "Decay Fit Parameter Map:X Resolution", "Decay Fit Parameter Map:Y Resolution", "Decay Fit Parameter Map:Use Decay Fit Result Constraints", "Decay Fit Parameter Map:Decay Fit Result Constraints", "Decay Fit Parameter Map:Decay Fit Result Constraints Applied", "---- Parameter Map ----", "Parameter Map:Palette Information", "Parameter Map:Palette List", "------- Local Decay Window ---------", "Local Decay Graph Window:Event Refnum", "Local Decay Graph Window:Use normalized IRF for convolution", "----- Miscellaneous ----", "Misc:Skippable Dialog Windows Status"}
  T48 = typedef "AlliGator Settings.lvlib/AlliGator Settings List.ctl" = enum16{"GUI:Visible Settings Tab", "GUI:Last Run Version", "Source Image:Use Image Histogram for Contrast", "Source Image:Low Count Pixels Rejection Options", "Source Image:High Count Pixels Rejection Options", "Source Image:Use Image Brightness", "Source Image:Blend Overlay with Image Background", "Source Image:Use Fixed ROI Diameter", "Source Image:ROI Diameter", "Source Image:ROI Center Color", "Source Image:Peak Threshold", "Source Image:Intensity Threshold", "Source Image:Image Binning Options", "Source Image:Image Smoothing Options", "Source Image:Image Histogram Active", "Source Image:Invert Binary Mask", "Source Image:Hot Pixel Removal", "Source Image:Overlay Analyzed ROI Center", "Source Image:Auto-Adjust Contrast", "Source Image:Histogram Lower Percentile", "Source Image:Histogram Upper Percentile", "Source Image:Save Source Image", "Source Image:Scale Bar Options", "Source Image:Image Resolution (Pixel Size)", "Source Image:Flatfield Correction", "Source Image:Show Dead Left Columns Correction", "Source Image:Dead Left Columns Correction", "Source Image:Image Pre-Processing Operations Order", "Source Image:Overlay ROI Median", "Source Image:Median Overlay Color", "Data Information:Gate Width", "Data Information:Nanotime Gate Separation", "Data Information:Macrotime Gate Separation", "Data Information:Gate Step", "Data Information:# Gates", "Data Information:Gate Image Exposure", "Data Information:Gate Image Integration", "Data Information:Gates to Skip", "Data Information:Gates to Keep", "Data Information:Define Gates to", "Data Information:Channel Name", "Data Information:Available Channel Names", "Data Information:Channel Arithmetic", "Data Information:Background File Subtraction", "Data Information:Background File", "Data Information:Background Scaling Factor", "Data Information:Background Pile-up Correction", "Data Information:Background Pixel Well Capacity", "Data Information:Laser Period", "Data Information:SYNC Period", "Data Information:Pile-up Correction", "Data Information:Pixel Well Capacity", "Data Information:Dataset Scaling Factor", "Fluorescence Decay_Decay Pre-Processing:Reverse Gates", "Fluorescence Decay_Decay Pre-Processing:Verbose Decay Pre-Processing", "Fluorescence Decay_Decay Pre-Processing:Use Decay Pre-Processing", "Fluorescence Decay_Decay Pre-Processing:Background Subtraction", "Fluorescence Decay_Decay Pre-Processing:Background Definition Range", "Fluorescence Decay_Decay Pre-Processing:Baseline Subtraction Method", "Fluorescence Decay_Decay Pre-Processing:Decay Pre-Processing Operations Order", "Fluorescence Decay_Decay Pre-Processing:Smoothing Parameter", "Fluorescence Decay_Decay Pre-Processing:Shift Decay", "Fluorescence Decay_Decay Pre-Processing:Decay Shift Parameters", "Fluorescence Decay_Decay Pre-Processing:Fold Decay", "Fluorescence Decay_Decay Pre-Processing:# Folds", "Fluorescence Decay_Decay Pre-Processing:1-Normalize Decay", "Fluorescence Decay_Decay Pre-Processing:[0-1]-Normalize Decay", "Fluorescence Decay_Decay Pre-Processing:Smoothen Decay", "Fluorescence Decay_Decay Pre-Processing:Extrapolate Decay", "Fluorescence Decay_Decay Pre-Processing:Use Periodicity", "Fluorescence Decay_Decay Pre-Processing:Use Cursors", "Fluorescence Decay_Decay Pre-Processing:Tail Fraction", "Fluorescence Decay_Decay Pre-Processing:Head Fraction", "Fluorescence Decay_Decay Pre-Processing:Additional Points", "Fluorescence Decay_Decay Pre-Processing:Straighten Decay", "Fluorescence Decay_Decay Pre-Processing:Constant Background", "Fluorescence Decay_Decay Pre-Processing:Pixel-Normalize Decay", "Fluorescence Decay_Advanced Analysis:Extract IRF instead of Decay", "Fluorescence Decay_Advanced Analysis:IRF Extraction Options", "Fluorescence Decay_Advanced Analysis:IRF Optimization Options", "Fluorescence Decay_Advanced Analysis:Square Pulse Options", "Fluorescence Decay_Advanced Analysis:IRF Order", "Fluorescence Decay_Advanced Analysis:IRF Time Constants", "Fluorescence Decay_Advanced Analysis:Wavelet Analysis Options", "Fluorescence Decay_Advanced Analysis:Average Lifetime Options", "Fluorescence Decay_Fit Options:Fit Options", "Fluorescence Decay_Fit Options:Use Legacy Fitting Approach", "Fluorescence Decay_Fit Options:Use Data Information Laser Period", "Fluorescence Decay_Fit Parameters:Displayed Fit Parameters", "Fluorescence Decay_Fit Parameters:Fit Parameter Constraints", "Fluorescence Decay_Fit Parameters:Export Tabulated Results", "Fluorescence Decay_Fit Parameters:MLE Baseline Offset Type", "Fluorescence Decay_Fit Parameters:MLE Baseline Offset", "Fluorescence Decay_Fit Parameters:Guess Parameter Names", "Fluorescence Decay_Fit Parameters:Guess Parameter Values", "Fluorescence Decay_Fit Parameters:Guess Parameters Options", "Fluorescence Decay_Fit Parameters:Optimal Offset Selection Criterion", "Fluorescence Decay_Styles:Show Last Decay Only", "Fluorescence Decay_Styles:Decay Graph Color Array", "Fluorescence Decay:Decay Graph Active", "Fluorescence Decay Statistics:Min Peak Value", "Fluorescence Decay Statistics:Reject Low Decay Peak Pixels", "Fluorescence Decay Statistics:Reject High Decay Peak Pixels", "Fluorescence Decay Statistics:Max Peak Value", "Time Traces:Use File Timestamp", "Time Traces:Time Step", "Time Traces:Use Intensity Correction File", "Time Traces:Intensity Correction File", "Phasor Plot:Phasor Plot Smoothing Options", "Phasor Plot:Phasor Plot Size", "Phasor Plot:Phasor Plot Graphics Options", "Phasor Plot:Cumulative Phasor Plot", "Phasor Plot:Use Phasor Brightness", "Phasor Plot:Blend Overlay with Phasor Background", "Phasor Plot:Save Phasor Plot", "Phasor Plot:Show References", "Phasor Plot:Phasor Ratio Decay Range", "Phasor Plot:Exponential Fading", "Phasor Plot:Phasor Ratio Reference Colors", "Phasor Plot:Reference Radius", "Phasor Plot:Show Color Map Vertices", "Phasor Plot:Phasor Plot Active", "Phasor Plot:Phasor Ratio Color Map Type", "Phasor Plot:Phasor Ratio Color Map", "Phasor Plot:Phasor Ratio Display Range", "Phasor Plot:Selected Image ROI(s)", "Phasor Plot:All Image ROIs", "Phasor Plot:Selected Phasor Plot ROI(s)", "Phasor Plot:All Phasor Plot ROIs", "Phasor Plot:Phasor Ratio Color-Coded Quantity", "Phasor Plot:Store Phasor Harmonics", "Phasor Plot:Draw Reference Segment", "Phasor Plot:User-Defined Quantity", "Phasor Plot:Color Scale High Color", "Phasor Plot:Color Scale Low Color", "Phasor Plot:Intensity-weighted Phasor Plot", "Phasor Graph:Phasor Frequency", "Phasor Graph:Phasor Ratio Type", "Phasor Graph:Pixel-level Phasor Computation", "Phasor Graph:Save Phasor Graph", "Phasor Graph:Phasor Graph Active", "Phasor Graph:Phasor SDV Options", "Phasor Graph:Intensity-weighted Phasor Graph", "Phasor Graph:Define Shortest Lifetime as", "Phasor Calibration:Use Backup Calibration if needed", "Phasor Calibration:Backup Calibration Type", "Phasor Calibration:Calibration Type", "Phasor Calibration:Calibration Lifetime", "Phasor Calibration:Calibration Map Algorithm", "Single-Exponential Phasor Locus (SEPL):Gate Parameters", "Single-Exponential Phasor Locus (SEPL):User-defined Gate", "Single-Exponential Phasor Locus (SEPL):User-defined IRF", "Single-Exponential Phasor Locus (SEPL):Phasor Parameters", "Single-Exponential Phasor Locus (SEPL):Decay & IRF Parameters", "Single-Exponential Phasor Locus (SEPL):Display Parameters", "Lifetime Analysis:Decay Analysis Parameters", "Lifetime Analysis:Lifetime Map Active", "Plugins:Python Settings", "Miscellaneous:Verbose Mode", "Miscellaneous:Beep after Script", "Miscellaneous:Saved Image File Format", "Miscellaneous:Exported Gate Image Settings", "Miscellaneous:Include Loading in Timing", "Miscellaneous:Verbose Settings Mode", "Miscellaneous:Histogram Options", "Miscellaneous:Beep on Error", "Miscellaneous:# Logical Processors Used", "Miscellaneous:ROI Description Max Characters", "Miscellaneous:Verbose Error Mode", "Miscellaneous:Transparent Mask Color"}
  T49 = typedef "AlliGator Internal Variables.lvlib/AlliGator Internal Variables v2.ctl" = cluster{"----------------------------- Images -----------------------------":u8, "Displayed Image":T50, "White Light Image":T50, "Mask Image":T50, "ROI Mask Image":T50, "Current Dataset Images 1":T51, "Background Dataset Images 1":T51, "Current Dataset Images 2":T51, "Background Dataset Images 2":T51, "Current Dataset Arithmetic Images":T51, "Accumulated Dataset Images 1":T51, "Accumulated Dataset Images 2":T51, "Accumulated Dataset Arithmetic Images":T51, "----------------------------- File Paths -----------------------------":u8, "Phasor Plot Image":T50, "Decay Fit Parameter Map Image":T50, "Parameter Map Image":T50, "Single Data Point Path":path, "White Light Image Path":path, "Mask Image Path":path, "Time-Series Folder":path, "[Time-Series Paths]":path[], "----------------------------- FLI Dataset -----------------------------":u8, "Current Dataset":i32, "Single Dataset Type":T23, "Current Folder":string, "AlliGator Data Series Type":T52, "# Datasets":i32, "Dual-Channel Dataset":bool, "Selected Channel Name":string, "Dataset Channel":T53, "Channel Arithmetic":T33, "Dual-Channel Background Dataset":bool, "Background Channel":T53, "Dual-Channel Accumulated Dataset":bool, "Start Time":dbl, "[Time-Series Timestamps]":dbl[], "[Intensity Corrections]":dbl[], "Time Series Script":bool, "Type of Displayed Image":T1, "Gate Image Slide":u16, "# Gates":i32, "ROIs":T54[], "----------------------------- Decays -----------------------------":u8, "ROI Decay":cluster{"t Array":dbl[], "I Array":dbl[]}, "Valid Decay":bool, "Decay  Metadata":T56, "Reference Decay Plot Name":string, "Reference Decay":cluster{"t Array":dbl[], "I Array":dbl[]}, "Decay Shift Plot":cluster{"Time Stamps":dbl[], "Decay Shifts":dbl[]}, "[Decays Max Values]":sgl[], "[Decays Min Values]":sgl[], "----------------------------- Calibration -----------------------------":u8, "Calibration Phasor":T59, "Calibration Phasor Series":T60, "Phasor Calibration Map":T61, "Calibration Map MD5 Digest":string, "----------------------------- Phasor Graph -----------------------------":u8, "Last Raw Phasor":T62, "Last Calibrated Phasor":T62, "Last Calibrated Phasor SDV":T62, "Phasor Graph:Phasor Plot":cluster{"g Array":dbl[], "s Array":dbl[]}, "Phasor Graph:Phasor SDV Plot":cluster{"g Array":dbl[], "s Array":dbl[]}, "[Phasor Graph:Raw Phasor Plots]":T63[], "Phasor Plot locked to Ref 1":i32, "[Phasor Plot(s) locked to Ref 1]":i32[], "[Phasor Plot(s) locked to Ref 2]":i32[], "[Pixel Phasors]":T62[], "----------------------------- Phasor Plot -----------------------------":u8, "[[Sum Image]]":dbl[][], "[[CSG Phasors]]":csg[][], "[[Valid Pixel?]]":bool[][], "[[Phasor Ratios]]":dbl[][], "[[Average Lifetimes]]":dbl[][], "Amplitude Weighted Average Lifetime":bool, "I/m/phi Dataset":cluster{"I/m/phi Dataset?":bool, "Base Frequency":dbl[unit], "Harmonic Orders":u8[]}, "Multi Phasor Plot Data":T65, "----------------------------- Decay Fit Parameter Map -----------------------------":u8, "Decay Fit Options & Parameters":T67, "Fit Options: Decay Preprocessing Parameters":T44, "Fit Options: Reference Decay":cluster{"t Array":dbl[], "I Array":dbl[]}, "Is Full Image Parameters Map":bool, "Is Single-Pixels Parameters Map":bool, "NLSF Parameters Map X Resolution":i32, "NLSF Parameters Map Y Resolution":i32, "[Single Decay Fit Parameters]":dbl[], "Fit Model":T69, "[[Multiple Decays Fit Parameters]]":dbl[][], "[[Multiple Decays Fit Parameter SDVs]]":dbl[][], "[[IRFs]]":dbl[][], "[ROI Descriptors]":T55[], "IRF Array Time Axis":dbl[], "Decay Array Time Axis":dbl[], "[Decay Fit Parameter Names]":T78[], "[Decay Sum]":dbl[], "Array of Decay Fit Result Constraints":T79[], "Selected ROIs Array":bool[], "----------------------------- Parameter Maps -----------------------------":u8, "[Map Set Names]":string[], "[Parameter Maps]":T80[], "[[User-defined Quantities]]":dbl[][], "User-defined Quantity":string}
  T50 = typedef "IMAQ Image.ctl" = refnum<image>
  T51 = typedef "AlliGator Internal Variables.lvlib/AlliGator Gate Image Set.ctl" = cluster{"SGL Gate Images":T50[], "SGL Sum Image":T50, "SGL Max Image":T50, "SGL Min Image":T50}
  T52 = typedef "AlliGator Files.lvlib/AlliGator Data Series Type.ctl" = enum16{"Not a Supported Series", "Gate Images Folder Series", "SwissSPAD 2 Dataset Series", "B&H FLI Dataset Series", "PicoQuant PTU FLI Dataset Series", "PicoQuant BIN FLI Dataset Series", "Piccolo hist BIN FLI Dataset Series", "HDF5 FLI Dataset Series"}
  T53 = typedef "AlliGator Dual-Channel Datasets.lvlib/AlliGator Dataset Channel.ctl" = enum16{"G2", "INT"}
  T54 = typedef "Image.lvlib/Named ROI Description.ctl" = cluster{"ROI Descriptor":T55, "ROI Name":string, "Overlay Color":u32}
  T55 = typedef "ROI Descriptor" = cluster{"Global Rectangle":i32[], "Contours":cluster{"ID":enum32{"External", "Internal"}, "Type":u32, "Coordinates":i32[]}[]}
  T56 = typedef "AlliGator Phasor Graph.lvlib/AlliGator Decay Metadata v3.ctl" = cluster{"ROI Descriptor":T55, "ROI Center":cluster{"X":i32, "Y":i32}, "Decay Background Subtraction Info":T57, "Decay Reverted":bool, "Decay Smoothened":bool, "Decay Straightened":bool, "Fitted Tau (Decay Straightening)":dbl, "Decay Shift Parameters":T45, "Decay Shifted":bool, "Decay Extrapolated":bool, "Decay Extrapolation Parameters":T58, "Decay Normalized":bool, "Fold Decay":bool, "# Folds":u32}
  T57 = typedef "AlliGator Decay Preprocessing.lvlib/AlliGator Decay Background Subtraction Info.ctl" = cluster{"Laser Period":dbl[unit], "Gate Duration":dbl[unit], "Baseline Subtraction Method":T43, "Background Definition Range":cluster{"Min Gate":dbl[unit], "Max Gate":dbl[unit]}, "Total Intensity w/o Bkgd Subtraction":dbl, "Bkgd-subtracted Intensity (exp)":dbl, "# Data Points":i32, "Background/Gate":dbl, "Fitted Lifetime":dbl[unit], "Bkgd-subtracted Intensity (theo)":dbl}
  T58 = typedef "AlliGator Decay Preprocessing.lvlib/AlliGator Decay Extrapolation Parameters.ctl" = cluster{"Additional Points":u32, "Head Fraction":dbl, "Fitted Tau":dbl, "Use Periodicity":bool, "Use Cursors":bool, "Tail Fraction":dbl}
  T59 = typedef "Phasor.lvlib/Calibration Phasor (m, phi).ctl" = cluster{"m":dbl, "phi":dbl, "Phasor Frequency":dbl[unit], "Reference Lifetime":dbl[unit]}
  T60 = typedef "Phasor.lvlib/Phasor Reference Series.ctl" = cluster{"m Array":dbl[], "phi Array":dbl[], "Phasor Frequency":dbl[unit], "Calibration Lifetime":dbl[unit]}
  T61 = typedef "Phasor.lvlib/Phasor Calibration Map v2.ctl" = cluster{"Phasor Frequency":dbl[unit], "Calibration Lifetime":dbl[unit], "ROI Centers":cluster{"X":i32, "Y":i32}[], "ROI Descriptors":T55[], "Map Resolution X":i32, "Map Resolution Y":i32, "z Array":cdb[]}
  T62 = typedef "Phasor.lvlib/Phasor (g, s).ctl" = cluster{"g":dbl, "s":dbl}
  T63 = typedef "AlliGator Phasor Graph.lvlib/AlliGator Raw Phasor Plot Data v5.ctl" = cluster{"Phasor Plot Name":string, "Raw Phasor Plot":T62[], "Phasor Frequency":dbl[unit], "[Decay Metadata]":T56[], "Raw Phasor Plot SDV":T62[], "Phasor SDV Options":T64, "[Calibration Phasor]":T59[], "Intensity Array":dbl[]}
  T64 = typedef "Phasor.lvlib/Phasor Standard Deviation Options.ctl" = cluster{"Compute Estimated SDV":bool, "# Replicas":u32, "Use Estimated Average Phasor":bool}
  T65 = typedef "AlliGator Phasor Plot.lvlib/AlliGator Phasor Multi-Harmonic Data.ctl" = cluster{"Base Frequency":dbl[unit], "# Harmonics":u8, "Harmonic Orders":u8[], "Phasor Plot Settings Checksum":u64, "Phasor Harmonic Data Array":T66[]}
  T66 = typedef "Phasor.lvlib/Phasor Harmonic Data.ctl" = cluster{"Phasor Harmonic Name":string, "Phasor Plot Settings Checksum":u64, "Phasor Frequency":dbl[unit], "Base Frequency":dbl[unit], "Harmonic Order":u8, "Phasor Plot Parameters":string, "Phasor Array [[CSG]]":csg[][], "Dataset File Path":path}
  T67 = typedef "AlliGator Decay Fit Parameter Map.lvlib/AlliGator Decay Fit Options & Parameters v4.ctl" = cluster{"SYNC Period":dbl[unit], "Fit Options":T68, "Fit Parameter Constraints":T75[], "MLE Baseline Offset":dbl, "MLE Baseline Offset Type":T77}
  T68 = typedef "Fits.lvlib/Decay Fit Options v4.ctl" = cluster{"Show Fit Residuals":bool, "Fit Model":T69, "Residual Type":T70, "Max Decay Percentile":dbl, "Min Decay Percentile":dbl, "Show Full Decay":bool, "Weights":T71, "Fitting Method":T72, "Compute Parameter Uncertainties":bool, "Periodic Boundaries":bool, "Model Calculation":T73, "Period":dbl[unit], "Termination Criteria":cluster{"Max Iterations":i32, "Max Function Calls":i32, "Max Time":dbl[unit], "Function Tolerance":dbl, "Parameter Tolerance":dbl, "Gradient Tolerance":dbl, "Min Lambda":dbl, "Max Lambda":dbl, "Initial Tick Count":u32}, "Offset Resolution":dbl[unit], "Use Local IRF":bool, "Fitting Algorithm":T74, "Show Confidence Interval ":bool, "Confidence Level":dbl}
  T69 = typedef "Fits.lvlib/Decay Model.ctl" = enum16{"1-Exponential", "2-Exponentials"}
  T70 = typedef "Fits.lvlib/Residual Type.ctl" = enum16{"Standard", "Normalized", "Reduced"}
  T71 = typedef "Fits.lvlib/Fit Weights Type v2.ctl" = enum16{"Unweighted", "1/Variance (Neyman)", "1/Variance (Pearson)", "Best of All"}
  T72 = typedef "Fits.lvlib/Non-linear Fitting Method v2.ctl" = enum16{"Least Square", "Least Absolute Residual", "Bisquare", "MLE", "-", "Best of All"}
  T73 = typedef "Fits.lvlib/Fit Calculation Method.ctl" = enum16{"Simulation", "Convolution", "Integration"}
  T74 = typedef "Fits.lvlib/Non-linear Fitting Algorithm.ctl" = enum16{"Levenberg-Marquardt", "Trust-Region Dogleg"}
  T75 = typedef "AlliGator Decay Fit.lvlib/AlliGator Decay Fit Parameter Constraints 2.ctl" = cluster{"Fit Parameter":T76, "Min Value":dbl, "Max Value":dbl, "Global":bool, "Used":bool}
  T76 = typedef "Fits.lvlib/Decay Fit Parameters In List.ctl" = enum16{"Offset", "Baseline", "A_1", "tau_1", "A_2", "tau_2"}
  T77 = typedef "Fits.lvlib/MLE Baseline Offset Type.ctl" = enum32{"Absolute", "Percentage"}
  T78 = typedef "Fits.lvlib/Decay Fit Parameters & Derived Quantities List v2.ctl" = enum16{"Offset", "Baseline", "A_1", "tau_1", "A_2", "tau_2", "<tau>_a", "f1_a", "f2_a", "<tau>_i", "f1_i", "f2_i", "-", "R^2", "Chi^2"}
  T79 = typedef "Fits.lvlib/Decay Fit Result Constraint.ctl" = cluster{"Fit Parameter":enum16{"Offset", "Baseline", "A_1", "tau_1", "A_2", "tau_2", "<tau>_a", "f1_a", "f2_a", "<tau>_i", "f1_i", "f2_i", "-", "R^2", "Chi^2", "Max Relative Residual", "<Residual ACF>", "Residual ACF SDV", "tau_2/tau_1"}, "Min Value":dbl, "Max Value":dbl, "Use Constraint":bool}
  T80 = typedef "AlliGator Decay Fit Parameter Map.lvlib/AlliGator Parameter Maps Data.ctl" = cluster{"Map Set Name":string, "[Parameter Names]":string[], "[[Parameters]]":dbl[][], "[[Parameter SDVs]]":dbl[][], "Decay Array Time Axis":dbl[], "[[IRFs]]":dbl[][], "IRF Array Time Axis":dbl[], "X Resolution":i32, "Y Resolution":i32, "Intensity Array":dbl[]}
  T81 = typedef "AlliGator Displayed Image.ctl" = enum16{"Single Gate", "Sum of All Gates", "Max of All Gates", "Min of All Gates", "-", "White Ligth Image", "Mask Image"}
  T82 = typedef "AlliGator Files.lvlib/AlliGator Batch File Conversion Item.ctl" = cluster{"File Path":path, "Saved":bool}
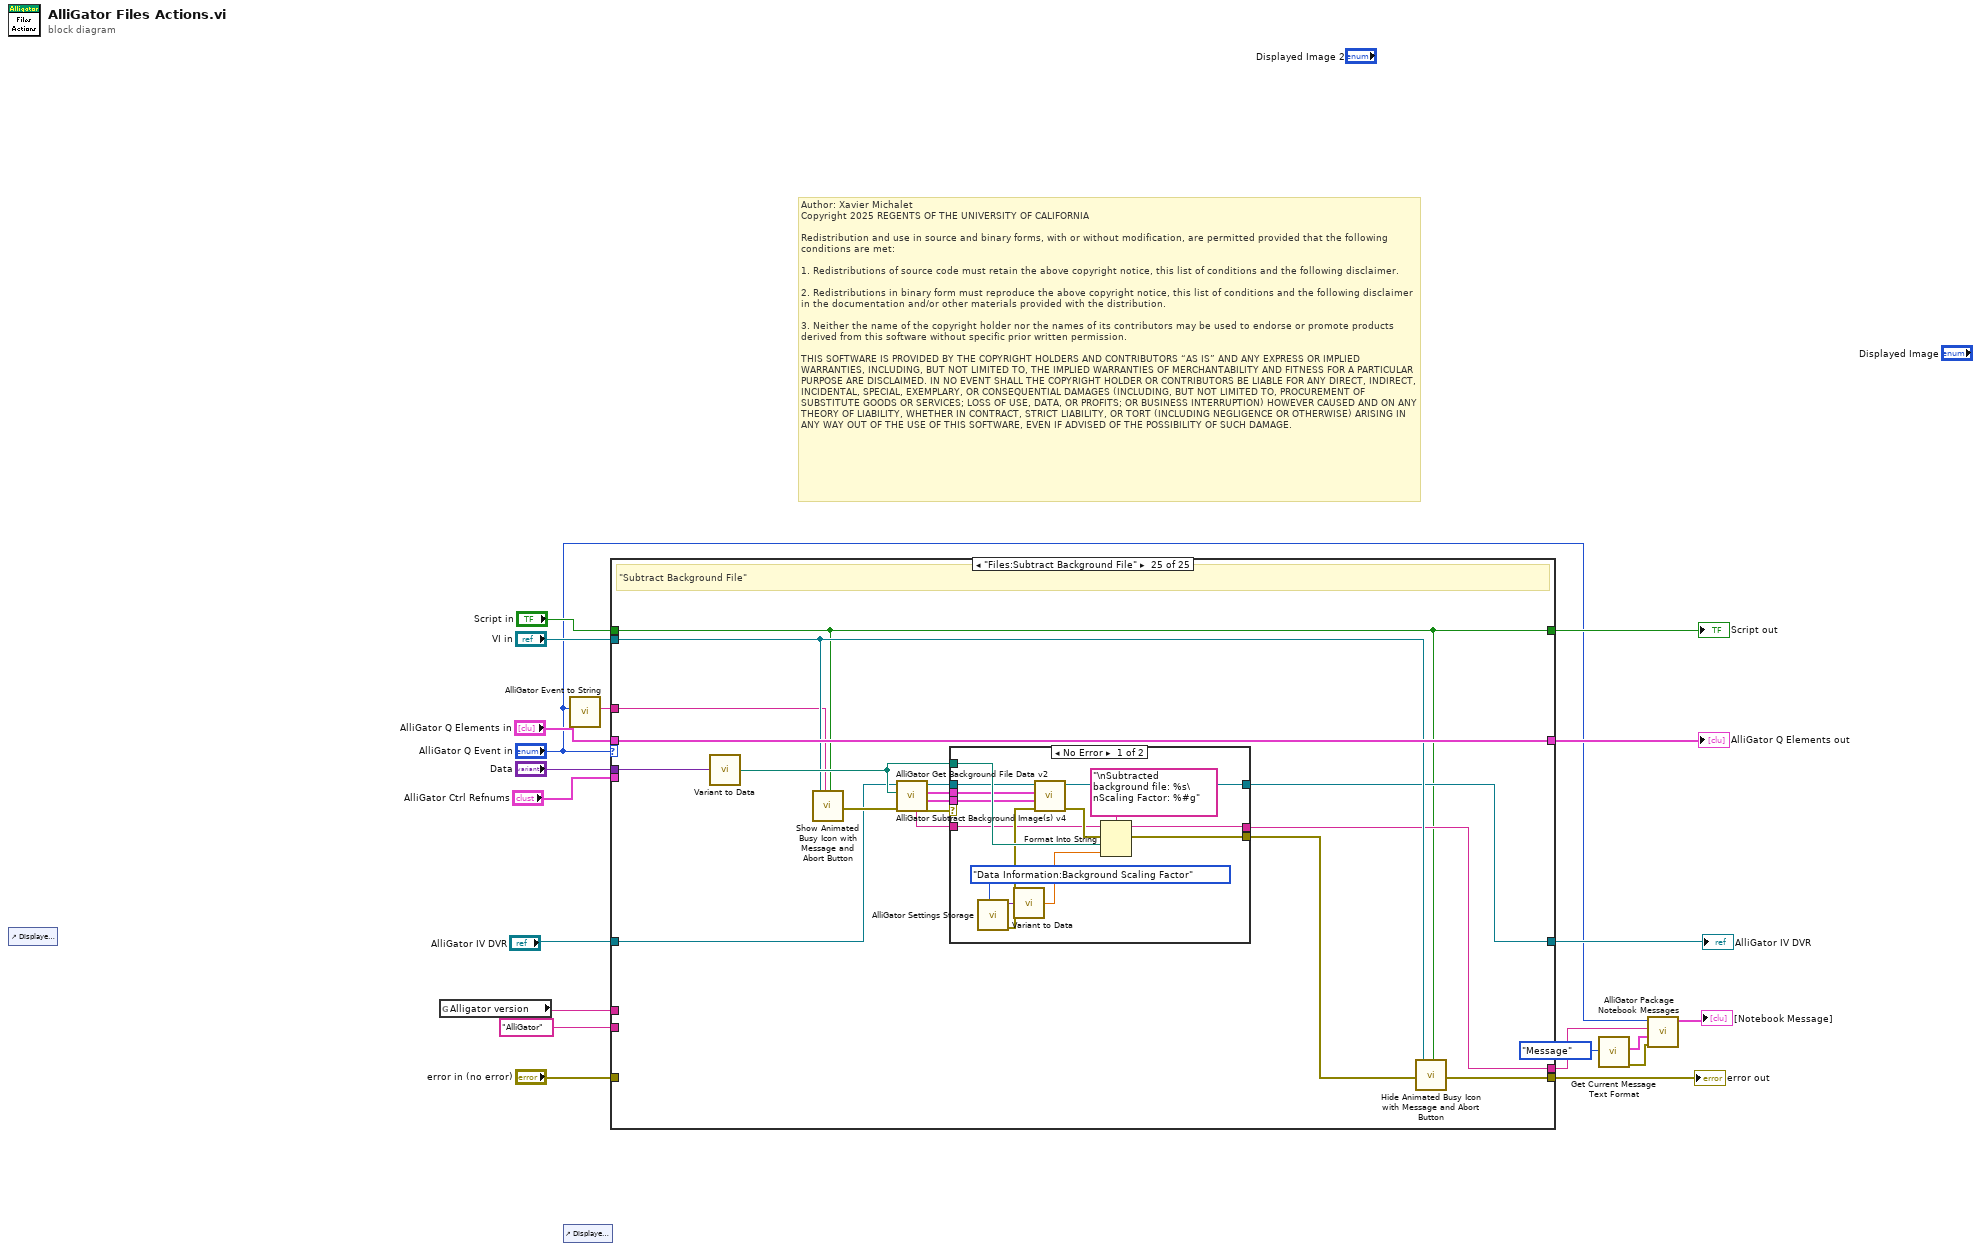
[diagram p0: block diagram]
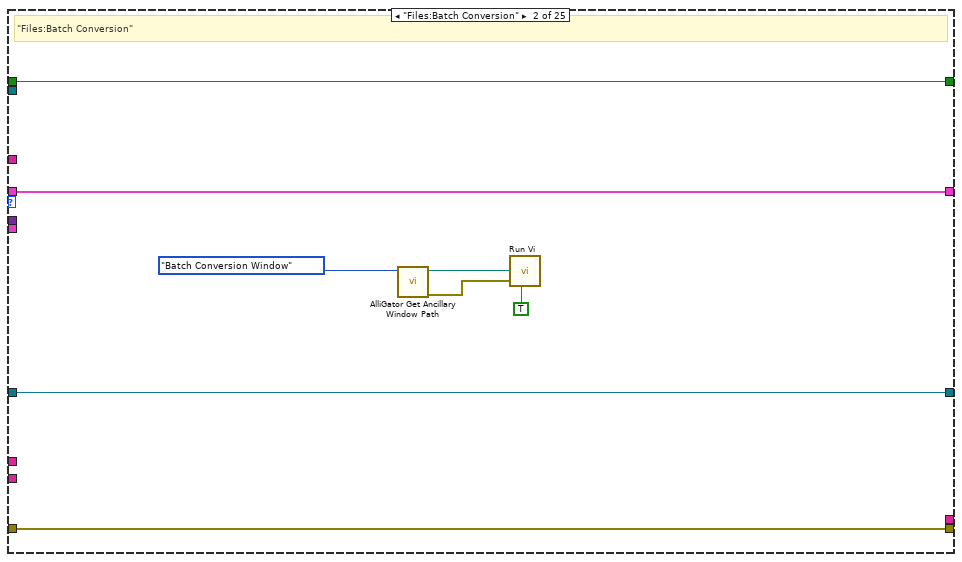
[diagram p3: hidden frame]
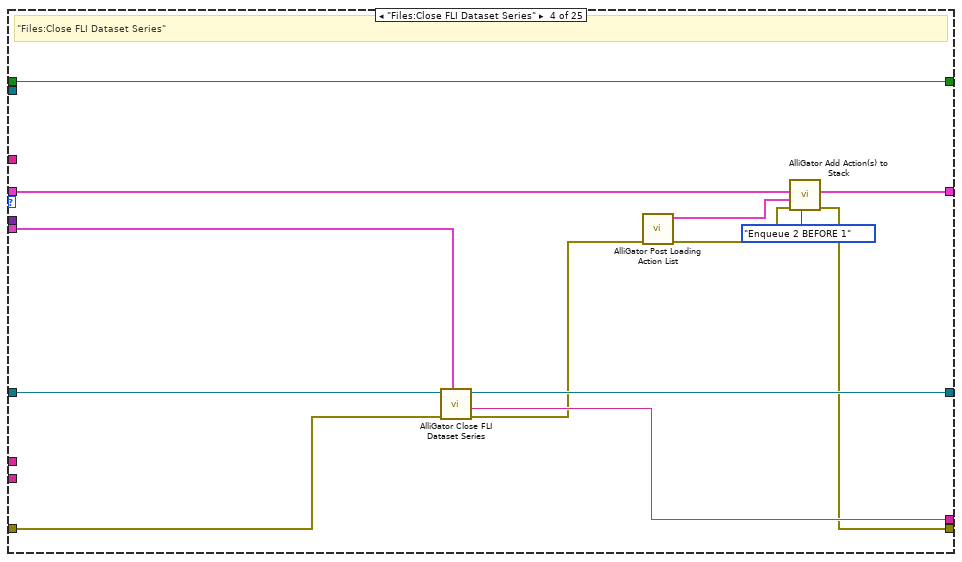
[diagram p5: hidden frame]
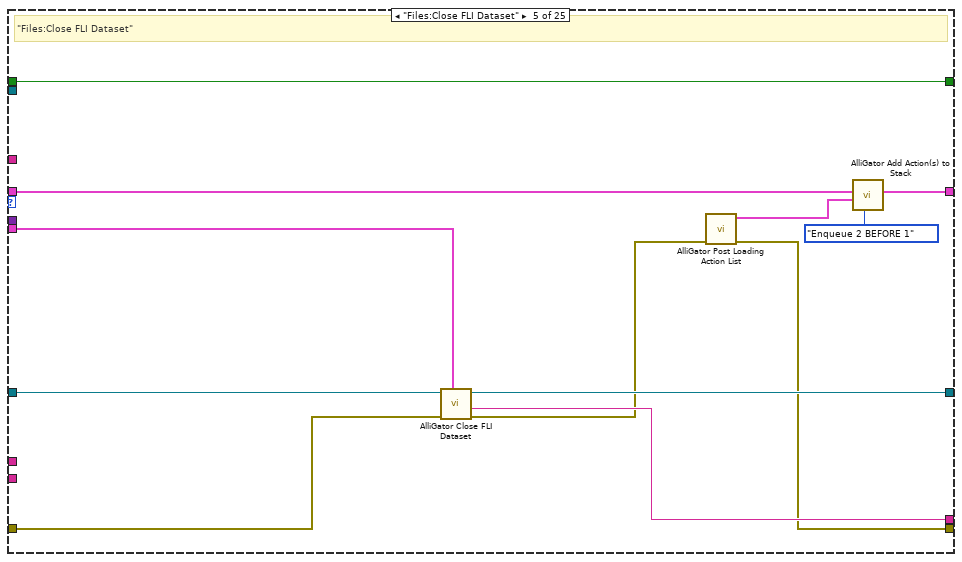
[diagram p6: hidden frame]
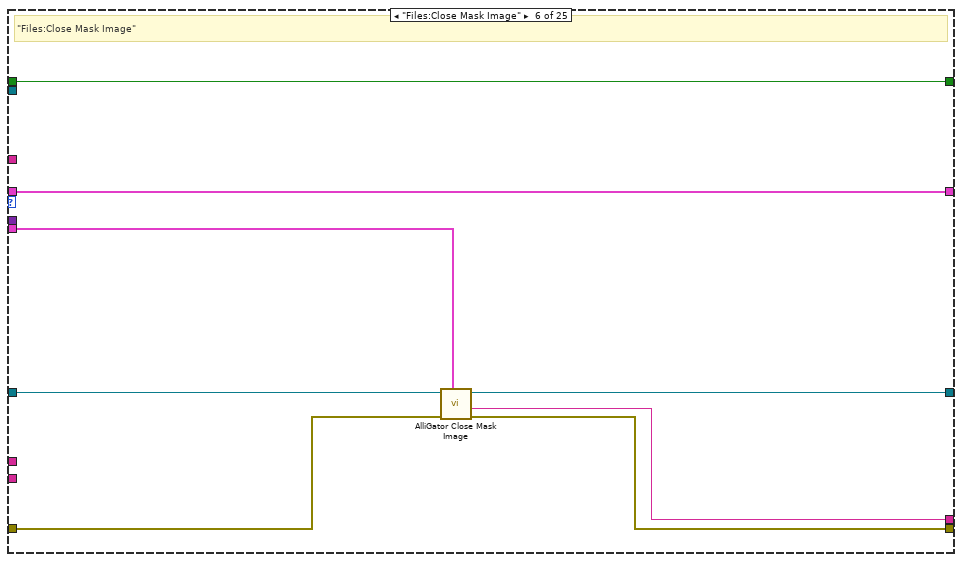
[diagram p7: hidden frame]
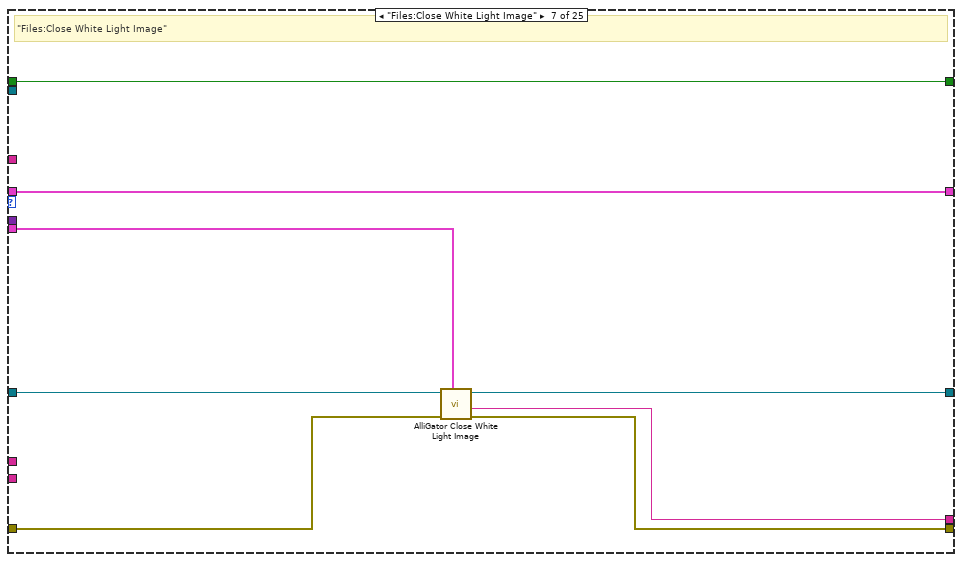
[diagram p8: hidden frame]
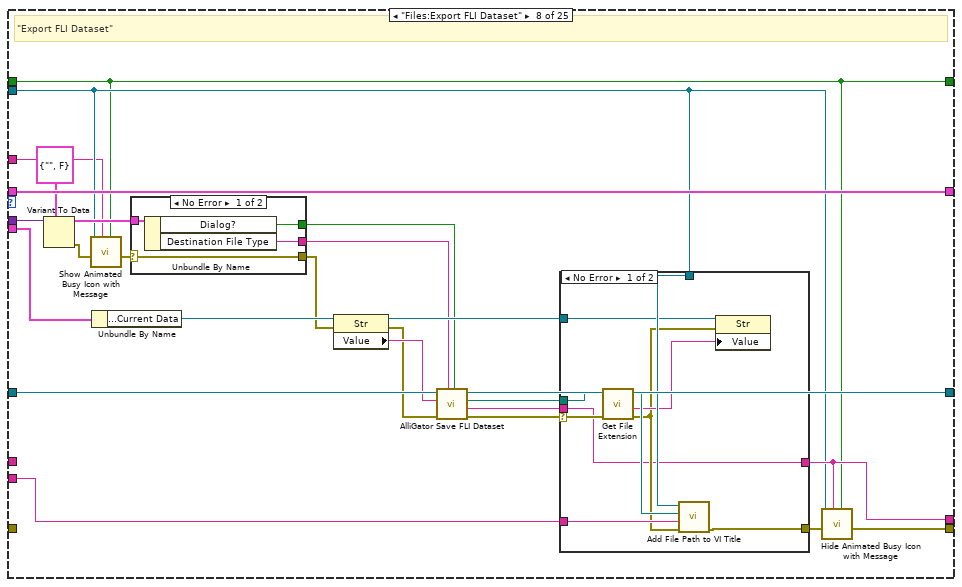
[diagram p9: hidden frame]
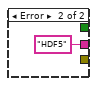
[diagram p10: hidden frame]
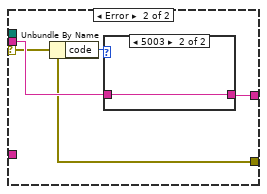
[diagram p11: hidden frame]
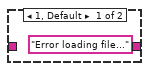
[diagram p12: hidden frame]
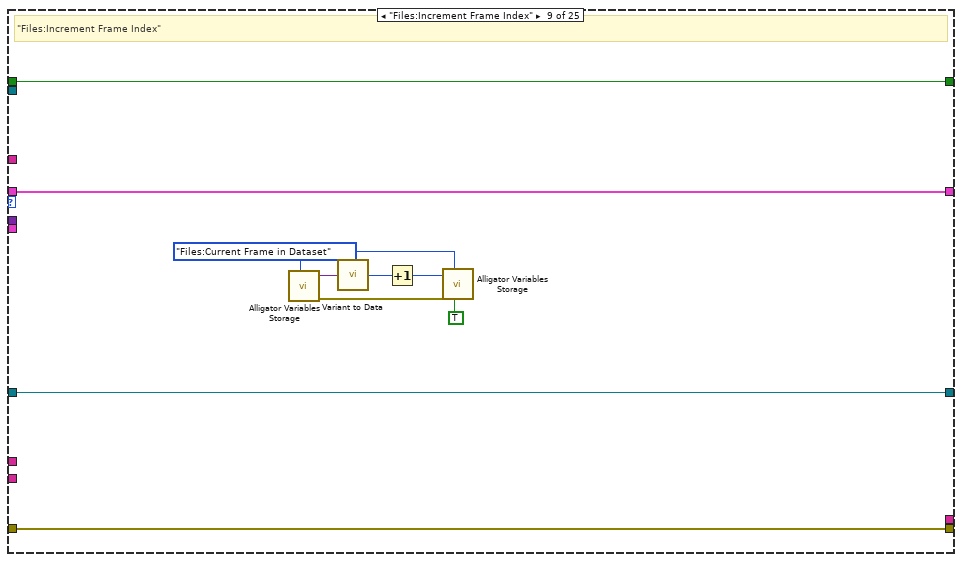
[diagram p13: hidden frame]
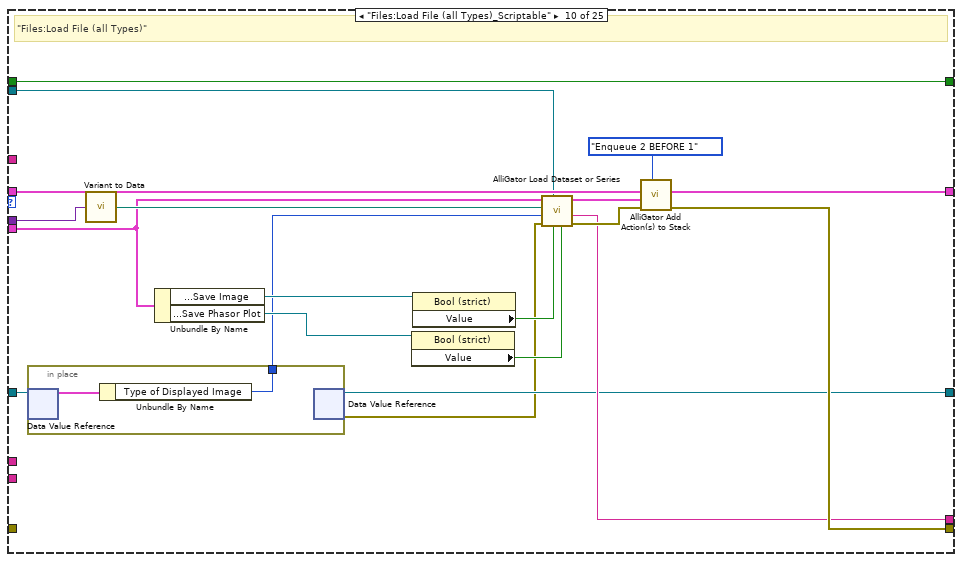
[diagram p14: hidden frame]
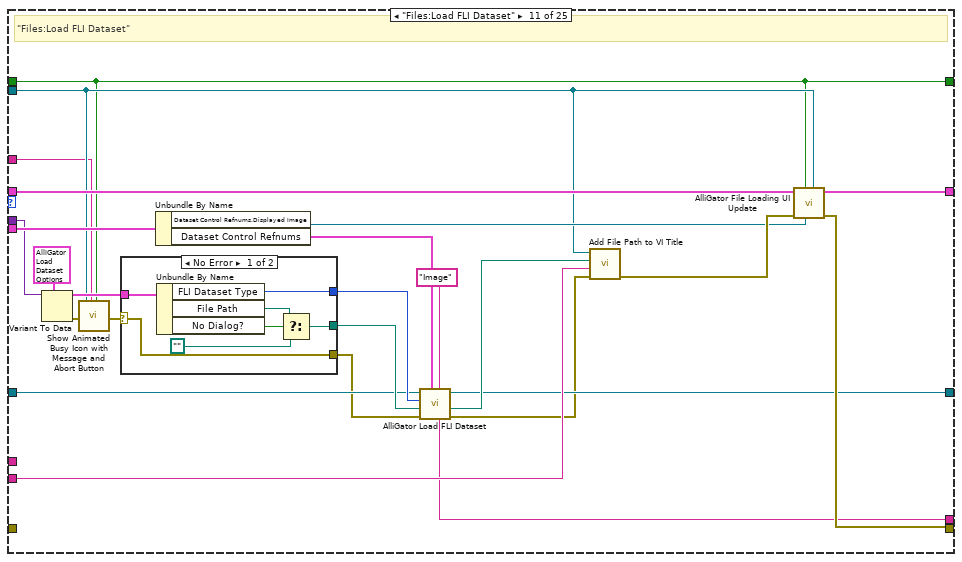
[diagram p15: hidden frame]
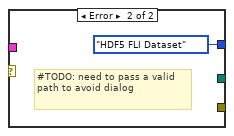
[diagram p16: hidden frame]
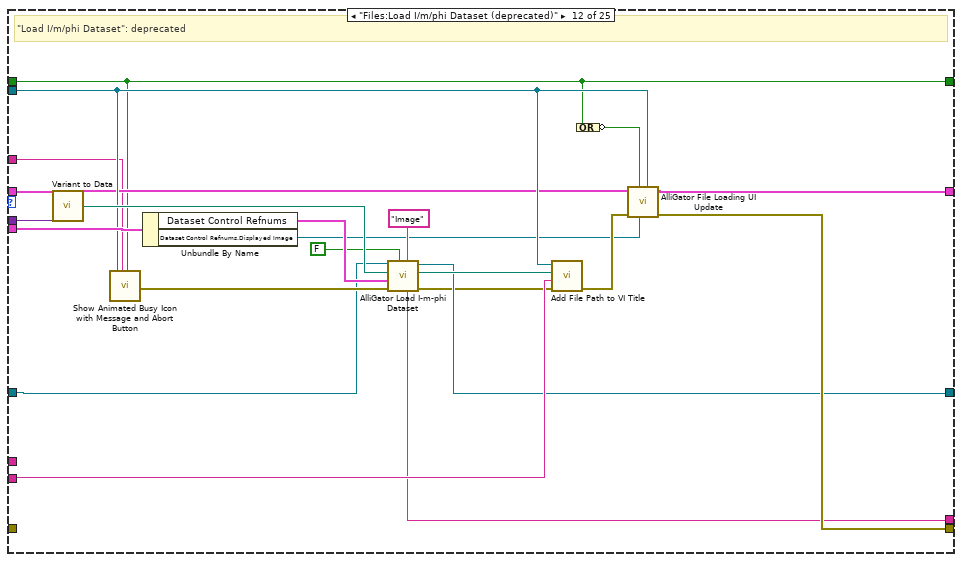
[diagram p17: hidden frame]
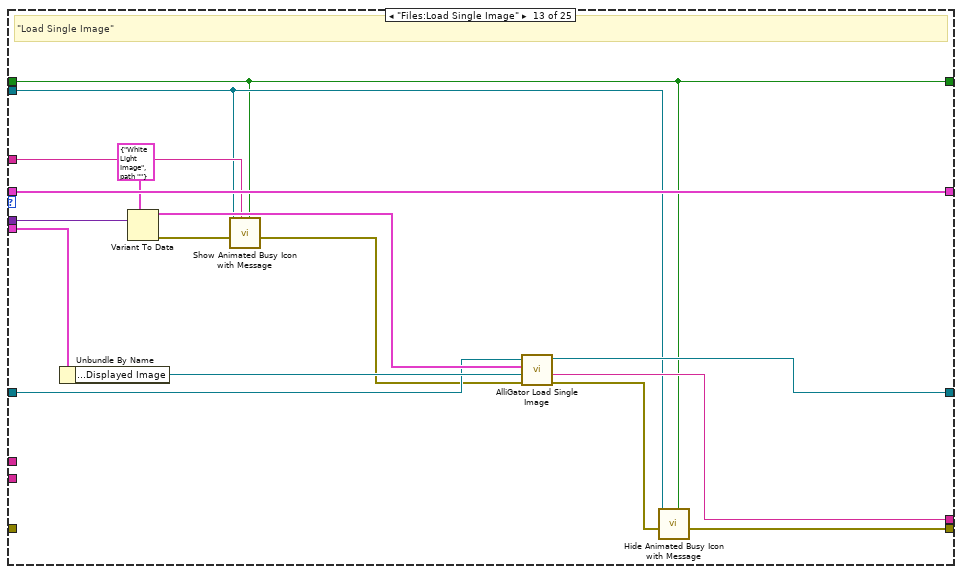
[diagram p18: hidden frame]
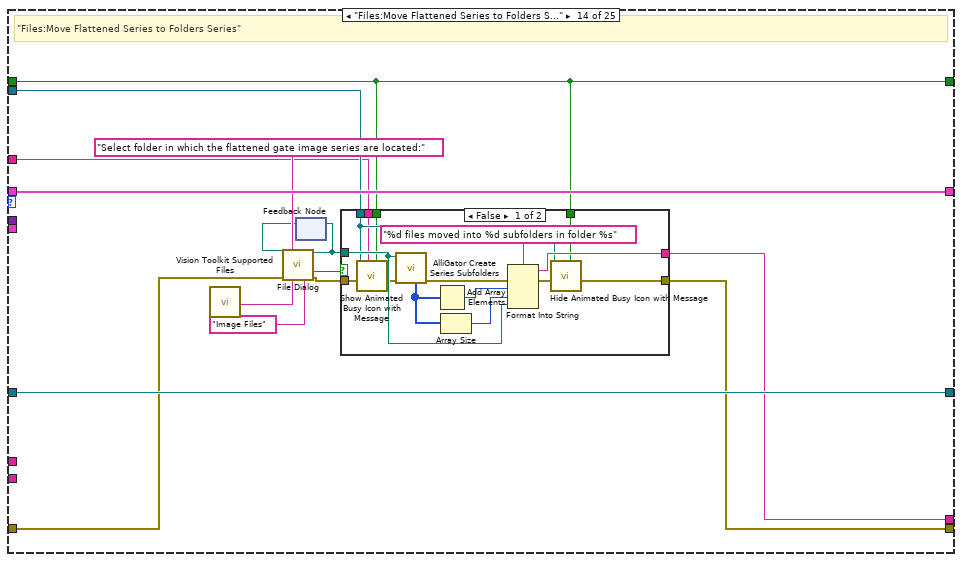
[diagram p19: hidden frame]
diagram:
  # "Author: Xavier Michalet\nCopyright 2025 REGENTS OF THE UNIVERSITY OF CALIFORNIA\n\nRedistribution and use in source and binary forms, with or without modification, are permitted provided that the following conditions are met:\n\n1. Redistributions of source code must retain the above copyright notice, this list of conditions and the following disclaimer.\n\n2. Redistributions in binary form must reproduce the above copyright notice, this list of conditions and the following disclaimer in the documentation and/or other materials provided with the distribution.\n\n3. Neither the name of the copyright holder nor the names of its contributors may be used to endorse or promote products derived from this software without specific prior written permission.\n\nTHIS SOFTWARE IS PROVIDED BY THE COPYRIGHT HOLDERS AND CONTRIBUTORS “AS IS” AND ANY EXPRESS OR IMPLIED WARRANTIES, INCLUDING, BUT NOT LIMITED TO, THE IMPLIED WARRANTIES OF MERCHANTABILITY AND FITNESS FOR A PARTICULAR PURPOSE ARE DISCLAIMED. IN NO EVENT SHALL THE COPYRIGHT HOLDER OR CONTRIBUTORS BE LIABLE FOR ANY DIRECT, INDIRECT, INCIDENTAL, SPECIAL, EXEMPLARY, OR CONSEQUENTIAL DAMAGES (INCLUDING, BUT NOT LIMITED TO, PROCUREMENT OF SUBSTITUTE GOODS OR SERVICES; LOSS OF USE, DATA, OR PROFITS; OR BUSINESS INTERRUPTION) HOWEVER CAUSED AND ON ANY THEORY OF LIABILITY, WHETHER IN CONTRACT, STRICT LIABILITY, OR TORT (INCLUDING NEGLIGENCE OR OTHERWISE) ARISING IN ANY WAY OUT OF THE USE OF THIS SOFTWARE, EVEN IF ADVISED OF THE POSSIBILITY OF SUCH DAMAGE."
  n1 = control-ref of="Displayed Image 2"() -> ()  [unwired: 1 out]
  n2 = global read "AlliGator Globals.vi" "Alligator version"() -> (w12:string)
  n3 = control-ref of="Displayed Image"() -> ()  [unwired: 1 out]
  n4 = call "AlliGator Event to String.vi"("AlliGator Q Event"="AlliGator Q Event in") -> ("String"=w8:string)  [unwired: 8 in]
  n5 = case shown="\"Files:Subtract Background File\"" "AlliGator Q Event in" {
    tunnel: "Data" -> [_ _ _ _ _ _ _ w99 _ w146 w173 w211 w227 _ _ w306 _ w380 _ _ w429 w460 w477 w485 w502]
    tunnel: "AlliGator Q Elements in" -> [w24 w32 w36 w41 w55 w69 w77 w103 w134 w153 w180 w197 w226 w242 w277 w308 w352 w375 w402 w415 w434 w463 w479 w487 w503]
    tunnel: [w24 w32 w36 w40 w54 w69 w77 w103 w134 w151 w179 w205 w226 w242 w275 w307 w350 w373 w400 w415 w433 w463 w479 w487 w503] -> w14
    tunnel: "VI in" -> [_ _ _ _ _ _ _ w82 _ w139 w160 w199 w213 w232 _ _ _ _ _ w407 w430 _ _ _ w496]
    tunnel: w12 -> [_ _ _ _ _ _ _ _ _ _ _ _ _ _ _ _ _ _ _ _ _ _ _ _ _]
    tunnel: [w23 w31 w35 w49 w61 w68 w76 w81 w133 w154 w159 w190 w212 w231 w279 w302 w353 w381 w404 w406 w431 w462 w478 w486 w489] -> w15
    tunnel: "Script in" -> [w23 w31 w35 w49 w61 w68 w76 w81 w133 w154 w159 w190 w212 w231 w279 w302 w353 w381 w404 w406 w431 w462 w478 w486 w489]
    tunnel: "AlliGator" ("Sender") -> [_ _ _ _ _ _ _ w102 _ _ w177 w202 _ _ _ _ _ _ _ _ w427 _ _ _ _]
    tunnel: "error in (no error)" -> [w22 w30 w34 w46 w58 w64 w72 _ w132 _ _ _ _ w234 _ _ _ _ _ w411 _ w461 _ _ _]
    tunnel: [w22 w30 w34 w39 w51 w65 w73 w101 w132 w149 w178 w204 w214 w235 w260 w287 w348 w371 w398 w408 w426 w461 w472 w481 w497] -> w1
    tunnel: "AlliGator Ctrl Refnums" -> [_ _ _ w45 w57 w63 w71 w100 _ w144 w176 w201 w223 _ w271 w296 _ w365 _ _ _ _ _ _ _]
    tunnel: "AlliGator IV DVR" -> [w21 w25 w33 w48 w60 w67 w75 w89 w131 w138 w166 w195 w220 w241 w261 w283 w346 w358 w396 w414 w420 w454 w471 w480 w493]
    tunnel: [w21 w25 w33 w47 w59 w66 w74 w86 w131 w137 w165 w194 w221 w241 w262 w282 w346 w357 w396 w413 w421 w454 w471 w480 w494] -> w9
    tunnel: w8 -> [_ _ _ _ _ _ _ w80 _ _ w158 w192 w215 w230 _ _ _ _ _ w409 _ _ _ _ w491]
    tunnel: [_ _ _ w44 w56 w62 w70 w98 _ w143 w163 w191 w217 w233 w259 w286 _ _ _ w405 _ _ _ _ w490] -> w6
    frame "---- Files ----", Default {
    }
    frame "Files:Batch Conversion" {
      # "\"Files:Batch Conversion\""
      n6 = call "AlliGator Get Ancillary Window Path.vi"("AlliGator Window"=AlliGator_Windows_List."Batch Conversion Window" ("AlliGator Windows")) -> ("Error Out"=w28:errorcluster, "VI Path"=w29:path)  [unwired: 9 in]
      n7 = call "Run Vi.vi"("VI Path"=w29, "error in (no error)"=w28, "Start Hidden? (F)"=TRUE) -> ()  [unwired: 5 in, 2 out]
    }
    frame "Files:Check #Frames in Dataset" {
      # "#TODO"
      # "\"Files:Check #Frames in Dataset\""
    }
    frame "Files:Close FLI Dataset Series" {
      # "\"Files:Close FLI Dataset Series\""
      n8 = call "AlliGator Close FLI Dataset Series.vi"("AlliGator Ctrl Refnums"=w45, "error in (no error)"=w46, "AlliGator IV DVR in"=w48) -> ("error out"=w38:errorcluster, "Message"=w44:string, "AlliGator IV DVR out"=w47:refnum<data-value>)  [unwired: 6 in]
      n9 = call "AlliGator Post Loading Action List.vi"("Error In"=w38) -> ("Error Out"=w37:errorcluster, "Action List"=w43:T7[])  [unwired: 9 in]
      n10 = call-poly "AlliGator Add Action(s) to Stack.vi"("Elements Order in Action Stack (Default: 2 BEFORE 1)"=Alligator_Elements_Order_in_Action_Stack."Enqueue 2 BEFORE 1", "Error In"=w37, "Alligator Queue Element 2"=w43, "Alligator Queue Element 1"=w41) -> ("Error Out"=w39:errorcluster, "Alligator Queue Element 1 (+ 2)"=w40:T7[])  [unwired: 6 in]
    }
    frame "Files:Close FLI Dataset" {
      # "\"Files:Close FLI Dataset\""
      n11 = call "AlliGator Close FLI Dataset.vi"("AlliGator Ctrl Refnums"=w57, "error in (no error)"=w58, "AlliGator IV DVR in"=w60) -> ("error out"=w52:errorcluster, "Message"=w56:string, "AlliGator IV DVR out"=w59:refnum<data-value>)  [unwired: 6 in]
      n12 = call "AlliGator Post Loading Action List.vi"("Error In"=w52) -> ("Error Out"=w51:errorcluster, "Action List"=w53:T7[])  [unwired: 9 in]
      n13 = call-poly "AlliGator Add Action(s) to Stack.vi"("Elements Order in Action Stack (Default: 2 BEFORE 1)"=Alligator_Elements_Order_in_Action_Stack."Enqueue 2 BEFORE 1", "Alligator Queue Element 2"=w53, "Alligator Queue Element 1"=w55) -> ("Alligator Queue Element 1 (+ 2)"=w54:T7[])  [unwired: 7 in, 1 out]
    }
    frame "Files:Close Mask Image" {
      # "\"Files:Close Mask Image\""
      n14 = call "AlliGator Close Mask Image.vi"("AlliGator Ctrl Refnums"=w63, "error in (no error)"=w64, "AlliGator IV DVR in"=w67) -> ("error out"=w65:errorcluster, "Message"=w62:string, "AlliGator IV DVR out"=w66:refnum<data-value>)  [unwired: 6 in]
    }
    frame "Files:Close White Light Image" {
      # "\"Files:Close White Light Image\""
      n15 = call "AlliGator Close White Light Image.vi"("AlliGator Ctrl Refnums"=w71, "error in (no error)"=w72, "AlliGator IV DVR in"=w75) -> ("error out"=w73:errorcluster, "Message"=w70:string, "AlliGator IV DVR out"=w74:refnum<data-value>)  [unwired: 6 in]
    }
    frame "Files:Export FLI Dataset" {
      # "\"Export FLI Dataset\""
      n16 = Variant To Data(type=T21 {"Destination File Type"="", "Dialog?"=FALSE} ("output cluster"), Variant=w99) -> (data=w92:T21, error out=w84:errorcluster)  [unwired: 1 in]
      n17 = call "Show Animated Busy Icon with Message.vi"("Already active? (F)"=w81, "Message"=w80, "Error In"=w84, "Target VI Refnum"=w82) -> ("Error Out"=w83:errorcluster)  [unwired: 7 in]
      n18 = Unbundle By Name(w100) -> ("Dataset Control Refnums.Current Data"=w93:refnum<vi>)
      n19 = case shown="No Error" w83 {
        selector: w83 -> [w104 _]
        tunnel: w92 -> [w107 _]
        tunnel: [w106 "HDF5" ("Destination File Type")] -> w88
        tunnel: [w105 _] -> w87
        tunnel: [w104 _] -> w79
        frame No Error {
          n20 = Unbundle By Name(w107) -> ("Dialog?"=w105:bool, "Destination File Type"=w106:string)
        }
        frame Error {
        }
      }
      n21 = property class="Str"(reference=w93, error in=w79) -> (reference out=w91:refnum<vi>, error out=w78:errorcluster, "Value"=w85:string)
      n22 = call "AlliGator Save FLI Dataset.vi"("Dialog?"=w87, "Destination File Type"=w88, "error in"=w78, "Current Data"=w85, "AlliGator IV DVR"=w89) -> ("error out"=w97:errorcluster, "Output String"=w95:string, "File Path out"=w94:path, "AlliGator IV DVR"=w86:refnum<data-value>)  [unwired: 3 in]
      n23 = case shown="No Error" w97 {
        selector: w97 -> [w114 w119]
        tunnel: [w113 w119] -> w96
        tunnel: w95 -> [w109 w122]
        tunnel: w94 -> [w117 _]
        tunnel: w82 -> [w118 _]
        tunnel: w102 -> [w116 _]
        tunnel: [w109 w120] -> w98
        tunnel: w91 -> [w112 _]
        frame No Error {
          n24 = call <vilib>:"Get File Extension.vi"("error in (no error)"=w114, "file"=w117) -> ("error out"=w110:errorcluster, "filename without extension"=w111:string, "dup file"=w115:path)  [unwired: 5 in, 2 out]
          n25 = call "Add File Path to VI Title.vi"("Error In"=w110, "VI Title"=w116, "File Path"=w115, "VI Refnum"=w118) -> ("Error Out"=w113:errorcluster)  [unwired: 7 in]
          n26 = property class="Str"(reference=w112, error in=w110, "Value"=w111) -> ()  [unwired: 2 out]
        }
        frame Error {
          n27 = Unbundle By Name(w119) -> ("code"=w121:i32)
          n28 = case shown="5003" w121 {
            tunnel: ["Error loading file..." ("Message") w124] -> w120
            tunnel: w122 -> [_ w124]
            frame 1, Default {
            }
            frame 5003 {
            }
          }
        }
      }
      n29 = call "Hide Animated Busy Icon with Message.vi"("Already active? (F)"=w81, "Message"=w98, "Error In"=w96, "Target VI reference"=w82) -> ("Error Out"=w101:errorcluster)  [unwired: 7 in]
    }
    frame "Files:Increment Frame Index" {
      w128 = AlliGator_Variables_List."Files:Current Frame in Dataset" ("Alligator Variable")
      # "\"Files:Increment Frame Index\""
      n30 = call "Alligator Variables Storage.vi"("AlliGator Variable"=w128) -> ("Error Out"=w129:errorcluster, "Data out"=w130:variant)  [unwired: 8 in, 1 out]
      n31 = call-poly "Variant to Data.vi"("Variant"=w130) -> ("Value"=w127:i32)  [unwired: 8 in]
      n32 = Increment(x=w127) -> (x+1=w126:i32)
      n33 = call "Alligator Variables Storage.vi"("Get(F)/Set"=TRUE, "AlliGator Variable"=w128, "Error In"=w129, "Data in"=w126) -> ()  [unwired: 5 in, 3 out]
    }
    frame "Files:Load File (all Types)_Scriptable" {
      # "\"Files:Load File (all Types)\""
      n34 = in-place {
        in-place-border: [w155] -> w135
        n35 = in-place-dvr #1(w138) -> (w156:T49)  [unwired: 1 out]
        n36 = Unbundle By Name(w156) -> ("Type of Displayed Image"=w155:T1)
        n37 = in-place-dvr #1() -> (w137:refnum<data-value>, w136:errorcluster)  [unwired: 1 in]
      }
      n38 = call-poly "Variant to Data.vi"("Variant"=w146) -> ("Path"=w145:path)  [unwired: 8 in]
      n39 = Unbundle By Name(w144) -> ("Dataset Control Refnums.Save Image"=w147:refnum<vi>, "Phasor Plot Ctrl Refnums.Save Phasor Plot"=w141:refnum<vi>)
      n40 = property class="Bool (strict)"(reference=w141) -> ("Value"=w140:bool)  [unwired: 1 in, 2 out]
      n41 = property class="Bool (strict)"(reference=w147) -> ("Value"=w142:bool)  [unwired: 1 in, 2 out]
      n42 = call "AlliGator Load Dataset or Series.vi"("Save Phasor Plot with Overlay"=w140, "Save Image with Overlay"=w142, "VI in"=w139, "error in (no error)"=w136, "Type of Displayed Image"=w135, "File/Folder Path"=w145, "AlliGator Ctrl Refnums"=w144) -> ("error out"=w150:errorcluster, "Message"=w143:string, "AlliGator Q Elements out"=w152:T7[])  [unwired: 2 in]
      n43 = call-poly "AlliGator Add Action(s) to Stack.vi"("Elements Order in Action Stack (Default: 2 BEFORE 1)"=Alligator_Elements_Order_in_Action_Stack."Enqueue 2 BEFORE 1", "Error In"=w150, "Alligator Queue Element 2"=w152, "Alligator Queue Element 1"=w153) -> ("Error Out"=w149:errorcluster, "Alligator Queue Element 1 (+ 2)"=w151:T7[])  [unwired: 6 in]
    }
    frame "Files:Load FLI Dataset" {
      # "\"Files:Load FLI Dataset\""
      n44 = Variant To Data(type=T22 {"FLI Dataset Type"=enum."HDF5 FLI Dataset", "No Dialog?"=FALSE, "File Path"=path ""} ("output cluster"), Variant=w173) -> (data=w172:T22, error out=w162:errorcluster)  [unwired: 1 in]
      n45 = call "Show Animated Busy Icon with Message and Abort Button.vi"("Already active? (F)"=w159, "Message"=w158, "Target VI reference"=w160, "Error In"=w162) -> ("Error Out"=w161:errorcluster)  [unwired: 15 in]
      n46 = case shown="No Error" w161 {
        selector: w161 -> [w182 _]
        tunnel: w172 -> [w188 _]
        tunnel: [w185 AlliGator_FLI_Dataset_Type."HDF5 FLI Dataset" ("FLI Dataset Type")] -> w170
        tunnel: [w183 _] -> w169
        tunnel: [w182 _] -> w157
        frame No Error {
          n47 = Unbundle By Name(w188) -> ("FLI Dataset Type"=w185:T23, "File Path"=w184:path, "No Dialog?"=w187:bool)
          n48 = Select(t=w184, s=w187, f=path "") -> (s? t:f=w183:path)
        }
        frame Error {
          # "#TODO: need to pass a valid path to avoid dialog"
        }
      }
      n49 = Unbundle By Name(w176) -> ("Dataset Control Refnums.Displayed Image"=w175:refnum<vi>, "Dataset Control Refnums"=w171:T13)
      n50 = call "AlliGator Load FLI Dataset.vi"("Image Type"="Image", "Dataset Control References"=w171, "error in"=w157, "Single Data Point Path"=w169, "FLI Dataset Type"=w170, "AlliGator IV DVR in"=w166) -> ("error out"=w164:errorcluster, "File Path out"=w168:path, "AlliGator IV DVR out"=w165:refnum<data-value>, "Message"=w163:string)  [unwired: 2 in]
      n51 = call "Add File Path to VI Title.vi"("Error In"=w164, "VI Title"=w177, "File Path"=w168, "VI Refnum"=w160) -> ("Error Out"=w181:errorcluster)  [unwired: 7 in]
      n52 = call "AlliGator File Loading UI Update.vi"("VI in"=w160, "Displayed Image"=w175, "Busy Icon already active?"=w159, "error in (no error)"=w181, "Alligator Queue Elements in"=w180) -> ("error out"=w178:errorcluster, "Alligator Queue Elements out"=w179:T7[])  [unwired: 5 in]
    }
    frame "Files:Load I/m/phi Dataset (deprecated)" {
      # "\"Load I/m/phi Dataset\": deprecated"
      n53 = call-poly "Variant to Data.vi"("Variant"=w211) -> ("Path"=w209:path)  [unwired: 8 in]
      n54 = call "Show Animated Busy Icon with Message and Abort Button.vi"("Already active? (F)"=w190, "Message"=w192, "Target VI reference"=w199) -> ("Error Out"=w208:errorcluster)  [unwired: 16 in]
      n55 = Unbundle By Name(w201) -> ("Dataset Control Refnums"=w200:T13, "Dataset Control Refnums.Displayed Image"=w198:refnum<vi>)
      n56 = call "AlliGator Load I-m-phi Dataset.vi"("Image Type"="Image", "Bkgd Image Subtraction?"=FALSE, "error in (no error)"=w208, "Control References"=w200, "Folder Path"=w209, "AlliGator IV DVR in"=w195) -> ("error out"=w193:errorcluster, "Folder Path (dup)"=w203:path, "AlliGator IV DVR out"=w194:refnum<data-value>, "Result String"=w191:string)  [unwired: 2 in]
      n57 = call "Add File Path to VI Title.vi"("Error In"=w193, "VI Title"=w202, "File Path"=w203, "VI Refnum"=w199) -> ("Error Out"=w206:errorcluster)  [unwired: 7 in]
      n58 = Compound Arithmetic op=OR(w190) -> (invert w207:bool)
      n59 = call "AlliGator File Loading UI Update.vi"("VI in"=w199, "Displayed Image"=w198, "Busy Icon already active?"=w207, "error in (no error)"=w206, "Alligator Queue Elements in"=w197) -> ("error out"=w204:errorcluster, "Alligator Queue Elements out"=w205:T7[])  [unwired: 5 in]
    }
    frame "Files:Load Single Image" {
      # "\"Load Single Image\""
      n60 = Unbundle By Name(w223) -> ("Dataset Control Refnums.Displayed Image"=w222:refnum<vi>)
      n61 = Variant To Data(type=T24 {"Image Type"=enum."White Light Image", "Image Path"=path ""}, Variant=w227) -> (data=w224:T24, error out=w218:errorcluster)  [unwired: 1 in]
      n62 = call "Show Animated Busy Icon with Message.vi"("Already active? (F)"=w212, "Message"=w215, "Error In"=w218, "Target VI Refnum"=w213) -> ("Error Out"=w216:errorcluster)  [unwired: 7 in]
      n63 = call "AlliGator Load Single Image.vi"("error in (no error)"=w216, "Displayed Image refnum"=w222, "Single Image File Info"=w224, "AlliGator Internal Data DVR"=w220) -> ("error out"=w219:errorcluster, "Message"=w217:string, "AlliGator Internal Data DVR"=w221:refnum<data-value>)  [unwired: 5 in]
      n64 = call "Hide Animated Busy Icon with Message.vi"("Already active? (F)"=w212, "Error In"=w219, "Target VI reference"=w213) -> ("Error Out"=w214:errorcluster)  [unwired: 8 in]
    }
    frame "Files:Move Flattened Series to Folders Series" {
      # "\"Files:Move Flattened Series to Folders Series\""
      n65 = call "Vision Toolkit Supported Files.vi"() -> ("Pattern String"=w239:string)  [unwired: 7 in, 1 out]
      n66 = feedback #2() -> (w229:path)  [unwired: 1 in]
      n67 = call "File Dialog"("start path"=w229, "prompt"="Select folder in which the flattened gate image series are located:", "error in"=w234, "pattern (all files)"=w239, "pattern label"="Image Files") -> ("selected path"=w228:path, "cancelled"=w236:bool, "error out"=w237:errorcluster)  [unwired: 7 in, 1 out]
      n68 = feedback-in #2(w228) -> ()
      n69 = case shown="False" w236 {
        tunnel: w228 -> [w249 _]
        tunnel: w237 -> [w257 w258]
        tunnel: [w247 w258] -> w235
        tunnel: [w254 _] -> w233
        tunnel: w232 -> [w246 _]
        tunnel: w231 -> [w245 _]
        tunnel: w231 -> [w244 _]
        tunnel: w230 -> [w243 _]
        frame False {
          n70 = call "Show Animated Busy Icon with Message.vi"("Already active? (F)"=w245, "Message"=w243, "Error In"=w257, "Target VI Refnum"=w246) -> ("Error Out"=w248:errorcluster)  [unwired: 7 in]
          n71 = call "AlliGator Create Series Subfolders.vi"("error in (no error)"=w248, "Path"=w249) -> ("error out"=w256:errorcluster, "# Files"=w252:i32[])  [unwired: 3 in, 5 out]
          n72 = Add Array Elements(numeric array=w252) -> (sum=w251:i32)
          n73 = Array Size(array=w252) -> (size(s)=w253:i32)
          n74 = Format Into String(format string="%d files moved into %d subfolders in folder %s", error in=w256, w251, w253, w249) -> (resulting string=w254:string, error out=w255:errorcluster)  [unwired: 1 in]
          n75 = call "Hide Animated Busy Icon with Message.vi"("Already active? (F)"=w244, "Error In"=w255, "Target VI reference"=w246) -> ("Error Out"=w247:errorcluster)  [unwired: 8 in]
        }
        frame True {
        }
      }
    }
    frame "Files:New Folder of Folders Selected" {
      w263 = TRUE ("Get(F)/Set")
      # "\"New Folder of Folders Selected\""
      n76 = Unbundle By Name(w271) -> ("Dataset Control Refnums.Time Point Slide"=w278:refnum<vi>, "Other AlliGator Ctrl Refnums.Use File Timestamp"=w267:refnum<vi>, "Dataset Control Refnums.Current Data"=w265:refnum<vi>, "Dataset Control Refnums.Time Point Slide"=w264:refnum<vi>)
      n77 = Unbundle By Name(w271) -> ("Phasor Plot Ctrl Refnums.Save Phasor Plot"=w272:refnum<vi>, "Dataset Control Refnums.Save Image"=w269:refnum<vi>)
      n78 = property class="Bool (strict)"(reference=w269) -> ("Value"=w268:bool)  [unwired: 1 in, 2 out]
      n79 = property class="Bool (strict)"(reference=w272) -> ("Value"=w270:bool)  [unwired: 1 in, 2 out]
      n80 = call "AlliGator Load First Dataset in FLI Dataset Series.vi"("Save Phasor Plot with Overlay"=w270, "Save Image with Overlay"=w268, "Time Slider Refnum"=w278, "AlliGator IV DVR in"=w261) -> ("Error Out"=w274:errorcluster, "Message"=w259:string, "AlliGator IV DVR out"=w262:refnum<data-value>, "Alligator Queue Elements out"=w276:T7[])  [unwired: 4 in]
      n81 = call-poly "AlliGator Add Action(s) to Stack.vi"("Elements Order in Action Stack (Default: 2 BEFORE 1)"=Alligator_Elements_Order_in_Action_Stack."Enqueue 2 BEFORE 1", "Error In"=w274, "Alligator Queue Element 2"=w276, "Alligator Queue Element 1"=w277) -> ("Error Out"=w260:errorcluster, "Alligator Queue Element 1 (+ 2)"=w275:T7[])  [unwired: 6 in]
      n82 = property class="Bool (strict)"(reference=w267, "Val(Sgnl)"=FALSE ("Value (Signaling)")) -> ()  [unwired: 1 in, 2 out]
      n83 = property class="Str"(reference=w265, "Visible"=w263) -> ()  [unwired: 1 in, 2 out]
      n84 = property class="Slide (strict)"(reference=w264, "Visible"=w263) -> ()  [unwired: 1 in, 2 out]
    }
    frame "Files:New Folder Selected" {
      # "\"New Folder Selected\""
      n85 = in-place {
        in-place-border: [w313] -> w290
        in-place-border: [w312] -> w289
        in-place-border: [w311] -> w288
        in-place-border: [w309] -> w280
        n86 = in-place-dvr #3(w283) -> (w310:T49)  [unwired: 1 out]
        n87 = Unbundle By Name(w310) -> ("Current Dataset"=w309:i32, "Single Data Point Path"=w313:path, "Single Dataset Type"=w312:T23, "[Time-Series Paths]"=w311:path[])
        n88 = in-place-dvr #3() -> (w282:refnum<data-value>, w281:errorcluster)  [unwired: 1 in]
      }
      n89 = Unbundle By Name(w296) -> ("Phasor Plot Ctrl Refnums.Save Phasor Plot"=w294:refnum<vi>, "Dataset Control Refnums.Save Image"=w292:refnum<vi>, "Dataset Control Refnums.Displayed Image"=w285:refnum<vi>)
      n90 = call-poly "Variant to Data.vi"("Variant"=w306) -> ("Path"=w305:path)  [unwired: 8 in]
      n91 = property class="Bool (strict)"(reference=w294) -> ("Value"=w293:bool)  [unwired: 1 in, 2 out]
      n92 = property class="Bool (strict)"(reference=w292) -> ("Value"=w291:bool)  [unwired: 1 in, 2 out]
      n93 = property class="Enum (strict)"(reference=w285) -> ("Value"=w284:T81)  [unwired: 1 in, 2 out]
      n94 = Empty Array?(array=w288) -> (empty?=w303:bool)
      n95 = call "AlliGator Update Data File.vi"("Error In"=w281, "Single Data Point Path"=w290, "New File Path in"=w305) -> ("Error Out"=w298:errorcluster, "Update Data File?"=w297:bool, "File Path out"=w300:path)  [unwired: 6 in]
      n96 = Path To String(path=w300) -> (string=w304:string)
      n97 = case shown="True" w297 {
        tunnel: w308 -> [w315 w322]
        tunnel: [w315 w321] -> w307
        tunnel: w300 -> [_ w328]
        tunnel: w298 -> [w314 w327]
        tunnel: w289 -> [_ w326]
        tunnel: w293 -> [_ w325]
        tunnel: w291 -> [_ w324]
        tunnel: [w314 w318] -> w295
        tunnel: w284 -> [_ w317]
        tunnel: w280 -> [_ w316]
        frame False {
        }
        frame True {
          n98 = call "AlliGator Script_Open Single FLI Dataset.vi"("Type of Displayed Image"=w317, "FLI Dataset Type"=w326, "File Path"=w328, "Dataset index in Series (0)"=w316, "Save Image with Overlay"=w325, "Error In"=w327, "Save Phasor Plot with Overlay"=w324) -> ("Action List out"=w323:T7[], "Error Out"=w319:errorcluster)  [unwired: 7 in]
          n99 = call-poly "AlliGator Add Action(s) to Stack.vi"("Elements Order in Action Stack (Default: 2 BEFORE 1)"=Alligator_Elements_Order_in_Action_Stack."Enqueue 2 BEFORE 1", "Error In"=w319, "Alligator Queue Element 2"=w323, "Alligator Queue Element 1"=w322) -> ("Error Out"=w318:errorcluster, "Alligator Queue Element 1 (+ 2)"=w321:T7[])  [unwired: 6 in]
        }
      }
      n100 = File/Directory Info(path=w300, error in=w295) -> (directory=w301:bool, error out=w299:errorcluster)  [unwired: 5 out]
      n101 = case shown="\"New Path\", Default" w304 {
        selector: w304 -> [_ w335]
        tunnel: w303 -> [_ w334]
        tunnel: w301 -> [_ w333]
        tunnel: w299 -> [w329 w332]
        tunnel: [w329 w331] -> w287
        tunnel: [_ w330] -> w286
        frame "" {
        }
        frame "New Path", Default {
          n102 = case shown="True" w334 {
            tunnel: w335 -> [_ w345]
            tunnel: w333 -> [_ w343]
            tunnel: w332 -> [w336 w339]
            tunnel: [w336 w337] -> w331
            tunnel: [_ w338] -> w330
            frame False {
            }
            frame True {
              n103 = Select(t="Folder" ("input 1"), s=w343, f="File" ("input 1")) -> (s? t:f=w341:string)
              n104 = Format Into String(format string="New %s Selected: %s" ("initial string"), error in=w339, w341, w345) -> (resulting string=w338:string, error out=w337:errorcluster)  [unwired: 1 in]
            }
          }
        }
      }
    }
    frame "Files:Open Mask Image" {
      # "\"Open Mask Image\""
      n105 = call "AlliGator Script Open Mask Image.vi"() -> ("Error Out"=w349:errorcluster, "Action List out"=w351:T7[])  [unwired: 10 in]
      n106 = call-poly "AlliGator Add Action(s) to Stack.vi"("Elements Order in Action Stack (Default: 2 BEFORE 1)"=Alligator_Elements_Order_in_Action_Stack."Enqueue 2 BEFORE 1", "Error In"=w349, "Alligator Queue Element 2"=w351, "Alligator Queue Element 1"=w352) -> ("Error Out"=w348:errorcluster, "Alligator Queue Element 1 (+ 2)"=w350:T7[])  [unwired: 6 in]
    }
    frame "Files:Open Single Dataset" {
      w362 = FALSE  # Single Dataset
      # "If loading fails, we lose this information!"
      # "\"Files:Open Single Dataset\""
      n107 = Unbundle By Name(w365) -> ("Dataset Control Refnums.Current Data"=w364:refnum<vi>, "Dataset Control Refnums.Time Point Slide"=w363:refnum<vi>)
      n108 = Variant To Data(type=T22 {"FLI Dataset Type"=enum."HDF5 FLI Dataset", "No Dialog?"=FALSE, "File Path"=path ""} ("output cluster"), Variant=w380) -> (data=w378:T22, error out=w356:errorcluster)  [unwired: 1 in]
      n109 = Unbundle By Name(w365) -> ("Phasor Plot Ctrl Refnums.Save Phasor Plot"=w369:refnum<vi>, "Dataset Control Refnums.Save Image"=w367:refnum<vi>, "Dataset Control Refnums.Displayed Image"=w360:refnum<vi>)
      n110 = case shown="Error .." w356 {
        selector: w356 -> [w390 _]
        tunnel: w378 -> [w393 _]
        tunnel: [w392 AlliGator_FLI_Dataset_Type."HDF5 FLI Dataset" ("FLI Dataset Type")] -> w377
        tunnel: [w391 TRUE ("No Dialog?")] -> w376
        tunnel: [w390 _] -> w355
        tunnel: [w389 _] -> w354
        frame No Error {
          n111 = Unbundle By Name(w393) -> ("No Dialog?"=w391:bool, "FLI Dataset Type"=w392:T23, "File Path"=w389:path)
        }
        frame Error {
          # "#TODO: pass dataset type"
        }
      }
      n112 = disable-structure shown="Enabled" {
        disable-tunnel: [w384 w387] -> w361
        disable-tunnel: w358 -> [w383 w388]
        disable-tunnel: [w382 w388] -> w357
        disable-tunnel: w354 -> [_ w387]
        frame Disabled {
          n113 = in-place {
            in-place-border: [w386] -> w384
            n114 = in-place-dvr #4(w383) -> (w385:T49)  [unwired: 1 out]
            n115 = Unbundle By Name(w385) -> ("Single Data Point Path"=w386:path)
            n116 = in-place-dvr #4() -> (w382:refnum<data-value>)  [unwired: 1 in, 1 out]
          }
        }
        frame Enabled {
        }
      }
      n117 = property class="Enum (strict)"(reference=w360) -> ("Value"=w359:T81)  [unwired: 1 in, 2 out]
      n118 = property class="Bool (strict)"(reference=w369) -> ("Value"=w368:bool)  [unwired: 1 in, 2 out]
      n119 = property class="Bool (strict)"(reference=w367) -> ("Value"=w366:bool)  [unwired: 1 in, 2 out]
      n120 = property class="Str"(reference=w364, "Visible"=w362) -> ()  [unwired: 1 in, 2 out]
      n121 = property class="Slide (strict)"(reference=w363, "Visible"=w362) -> ()  [unwired: 1 in, 2 out]
      n122 = call "AlliGator Script_Open Single FLI Dataset.vi"("Type of Displayed Image"=w359, "FLI Dataset Type"=w377, "No Dialog? (T)"=w376, "File Path"=w361, "Save Image with Overlay"=w368, "Error In"=w355, "Save Phasor Plot with Overlay"=w366) -> ("Action List out"=w374:T7[], "Error Out"=w372:errorcluster)  [unwired: 7 in]
      n123 = call-poly "AlliGator Add Action(s) to Stack.vi"("Elements Order in Action Stack (Default: 2 BEFORE 1)"=Alligator_Elements_Order_in_Action_Stack."Enqueue 2 BEFORE 1", "Error In"=w372, "Alligator Queue Element 2"=w374, "Alligator Queue Element 1"=w375) -> ("Error Out"=w371:errorcluster, "Alligator Queue Element 1 (+ 2)"=w373:T7[])  [unwired: 6 in]
    }
    frame "Files:Open White Light Image" {
      # "\"Open Single Image\""
      n124 = call "AlliGator Script Open White Light Image.vi"("Image Path"=path "") -> ("Error Out"=w399:errorcluster, "Action List out"=w401:T7[])  [unwired: 9 in]
      n125 = call-poly "AlliGator Add Action(s) to Stack.vi"("Elements Order in Action Stack (Default: 2 BEFORE 1)"=Alligator_Elements_Order_in_Action_Stack."Enqueue 2 BEFORE 1", "Error In"=w399, "Alligator Queue Element 2"=w401, "Alligator Queue Element 1"=w402) -> ("Error Out"=w398:errorcluster, "Alligator Queue Element 1 (+ 2)"=w400:T7[])  [unwired: 6 in]
    }
    frame "Files:Save Mask Image" {
      # "\"Files:Save Mask Image\""
      n126 = call "Show Animated Busy Icon with Message.vi"("Already active? (F)"=w406, "Message"=w409, "Error In"=w411, "Target VI Refnum"=w407) -> ("Error Out"=w410:errorcluster)  [unwired: 7 in]
      n127 = call "AlliGator Save Mask Image.vi"("error in (no error)"=w410, "AlliGator IV DVR in"=w414) -> ("error out"=w412:errorcluster, "Message"=w405:string, "AlliGator IV DVR out"=w413:refnum<data-value>)  [unwired: 7 in]
      n128 = call "Hide Animated Busy Icon with Message.vi"("Already active? (F)"=w406, "Message"=w405, "Error In"=w412, "Target VI reference"=w407) -> ("Error Out"=w408:errorcluster)  [unwired: 7 in]
    }
    frame "Files:Select Folder" {
      # "\"Select Folder\""
      n129 = Variant To Data(type=T26 {"Folder Selection Mode"=enum."Select Gate Folder", "Folder Path"=path ""} ("Folder Selection"), Variant=w429) -> (data=w423:T26, error out=w417:errorcluster)  [unwired: 1 in]
      n130 = case shown="Error .." w417 {
        selector: w417 -> [w435 _]
        tunnel: w423 -> [w438 _]
        tunnel: [w437 _] -> w422
        tunnel: [w436 AlliGator_Select_Folder_Mode."Select Folder of HDF5 FLI Datasets" ("Folder Selection Mode")] -> w418
        tunnel: [w435 _] -> w416
        frame No Error {
          n131 = Unbundle By Name(w438) -> ("Folder Path"=w437:path, "Folder Selection Mode"=w436:T27)
        }
        frame Error {
          # "#TODO: pass folder path and type"
        }
      }
      n132 = call "AlliGator Select Folder.vi"("Error In"=w416, "Folder Selection Mode"=w418, "Folder Path"=w422, "AlliGator IV DVR in"=w420) -> ("Error Out"=w419:errorcluster, "cancelled"=w432:bool, "selected path"=w428:path, "AlliGator IV DVR out"=w421:refnum<data-value>, "AlliGator Q Element"=w425:T7)  [unwired: 3 in]
      n133 = case shown="True" w432 {
        tunnel: w434 -> [w448 w452]
        tunnel: [w447 w452] -> w433
        tunnel: w425 -> [w444 _]
        tunnel: w430 -> [w445 _]
        tunnel: w428 -> [w442 _]
        tunnel: w427 -> [w443 _]
        tunnel: w419 -> [w441 w451]
        tunnel: [w440 w450] -> w426
        frame False {
          n134 = call "Add File Path to VI Title.vi"("Error In"=w441, "VI Title"=w443, "File Path"=w442, "VI Refnum"=w445) -> ("Error Out"=w440:errorcluster)  [unwired: 7 in]
          n135 = call-poly "AlliGator Add Action(s) to Stack.vi"("Elements Order in Action Stack (Default: 2 BEFORE 1)"=Alligator_Elements_Order_in_Action_Stack."Enqueue 2 BEFORE 1", "Alligator Atomic Action"=w444, "Alligator Queue Element 1"=w448) -> ("Alligator Queue Element 1 (+ 2)"=w447:T7[])  [unwired: 7 in, 1 out]
        }
        frame True {
          w449 = 43  # Operation cancelled by user
          n136 = call <vilib>:"Clear Errors.vi"("error in (no error)"=w451, "specific error code to clear (0: all)"=w449) -> ("error out"=w450:errorcluster)  [unwired: 4 in, 1 out]
        }
      }
    }
    frame "Files:Set Batch Export Files To Save" {
      # "\"Set Batch Export File To Save\""
      n137 = call-poly "Variant to Data.vi"("Variant"=w460) -> ("Path"=w457:path)  [unwired: 8 in]
      n138 = call "AlliGator Batch Export Status.vi"("Set/Get (F)"=FALSE) -> ("error out"=w453:errorcluster, "Conversion Jobs out"=w458:T82[])  [unwired: 9 in]
      n139 = for {
        tunnel: w458 -> [w468] mode=indexing
        tunnel: w457 -> [w469]
        tunnel: [w465] -> w456 mode=indexing
        n140 = Unbundle By Name(w468) -> ("File Path"=w470:path, "Saved"=w467:bool)
        n141 = Equal?(x=w469, y=w470) -> (x = y?=w466:bool)
        n142 = Or(x=w466, y=w467) -> (x .or. y?=w464:bool)
        n143 = Bundle By Name(cluster=w468, "Saved"=w464) -> (w465:T82)
      }
      n144 = call "AlliGator Batch Export Status.vi"("Set/Get (F)"=TRUE, "error in (no error)"=w453, "Conversion Jobs in"=w456) -> ()  [unwired: 7 in, 2 out]
    }
    frame "Files:Set Dataset Loading & Pre-processing Options" {
      # "\"Set Dataset Loading & Pre-processing Options\""
      n145 = Variant To Data(type=T28 {"Data Information"={"Gates to Skip"={"Start"=0, "End"=0}, "# Gates"=1, "Gate Step"=1, "Gate Duration"=3e-10, "Gate Separation"=4e-11, "Pile-up Correction"=FALSE, "Pixel Well Capacity"=1, "Define Gates to"=enum."Skip", "Gates to Keep"={"First"=0, "Last"=0}, "Laser Period"=0.0, "SYNC Period"=0.0, "Channel Name"=0, "Channel Arithmetic"=enum."None", "Background File Subtraction"=FALSE, "Background Scaling Factor"=1.0, "Background File"=path "", "Background Pile-up Correction"=FALSE, "Background Pixel Well Capacity"=1, "Dataset Scaling Factor"=1.0}, "Source Image Settings"={"Low Count Pixels Rejection Options"={"Background Low Threshold Factor"=0.0, "Fixed Low Background Threshold"=20000.0, "Reject Low Count Pixels"=FALSE, "Low Percentile"=0.0}, "High Count Pixels Rejection Options"={"Background High Threshold Factor"=0.0, "Fixed High Background Threshold"=1.0, "Reject High Count Pixels"=FALSE, "High Percentile"=100.0}, "Peak Threshold"=500.0, "Intensity Threshold"=500.0, "Image Smoothing Options"={"Use Image Smoothing"=FALSE, "Kernel Type"=enum."Bilinear", "Bin"=1, "Algorithm"=enum."Rapid"}, "Image Binning Options"={"Use Image Binning"=FALSE, "X Bin"=1, "Y Bin"=1}}, "Decay Preprocessing Options & Parameters"={"Background Subtraction Parameters"={"Background Definition Range"={"Min Gate"=0.0, "Max Gate"=0.0}, "Baseline Subtraction Method"=enum."Mean", "Background Subtraction?"=FALSE, "Background File"=path "", "Background Constant"=0.0, "Background Scaling Factor"=1.0, "Background Pile-up Correction"=FALSE, "Background Pixel Well Capacity"=1}, "Decay Preprocessing Parameters"={"Background Subtraction"=FALSE, "Straighten Decay"=FALSE, "Reverse Gates"=FALSE, "1-Normalized Decay"=FALSE, "Smoothen Decay"=FALSE, "Smoothing Parameter"=0.0, "Shift Decay"=FALSE, "Decay Shift Parameters"={"Type"=enum."Default", "Shift"=0.0, "Threshold"=0.0, "Rotate"=FALSE}, "Extrapolate Decay"=FALSE, "Additional Points"=0, "Head Fraction"=0.0, "Pixel-Normalize Decay"=FALSE, "Use Periodicity"=FALSE, "Use Cursors"=FALSE, "Tail Fraction"=0.0, "Use Decay Pre-Processing"=TRUE, "Fold Decay"=FALSE, "# Folds"=1, "[0-1]-Normalized Decay"=FALSE}, "Preprocessing Steps Order"=[]}, "Clear Phasor Graph"=FALSE} ("Dataset Loading & Pre-processing Options"), Variant=w477) -> (data=w475:T28, error out=w474:errorcluster)  [unwired: 1 in]
      n146 = call "AlliGator Get-Set Loading & Pre-Processing Options.vi"("Get (F)/Set"=TRUE, "Error In"=w474, "Dataset Loading & Pre-processing Options (in)"=w475) -> ("Error Out"=w472:errorcluster)  [unwired: 7 in, 1 out]
    }
    frame "Files:Set Destination File Path" {
      # "\"Set Destination File Path\""
      n147 = call-poly "Variant to Data.vi"("Variant"=w485) -> ("Path"=w484:path)  [unwired: 8 in]
      n148 = call "Alligator Variables Storage.vi"("Get(F)/Set"=TRUE, "AlliGator Variable"=AlliGator_Variables_List."Destination File Path" ("Alligator Variable"), "Data in"=w484) -> ("Error Out"=w481:errorcluster)  [unwired: 6 in, 2 out]
    }
    frame "Files:Subtract Background File" {
      # "\"Subtract Background File\""
      n149 = call-poly "Variant to Data.vi"("Variant"=w502) -> ("Path"=w498:path)  [unwired: 8 in]
      n150 = call "Show Animated Busy Icon with Message and Abort Button.vi"("Already active? (F)"=w489, "Message"=w491, "Target VI reference"=w496) -> ("Error Out"=w495:errorcluster)  [unwired: 16 in]
      n151 = call "AlliGator Get Background File Data v2.vi"("Error In"=w495, "Path"=w498, "AlliGator IV DVR in"=w493) -> ("Error Out"=w504:errorcluster, "Background Gate Images, Max & Sum 2"=w499:T51, "Background Gate Images, Max & Sum 1"=w500:T51, "AlliGator IV DVR out"=w501:refnum<data-value>, "Message"=w488:string)  [unwired: 4 in]
      n152 = case shown="No Error" w504 {
        selector: w504 -> [_ w521]
        tunnel: w501 -> [w512 w520]
        tunnel: w500 -> [w510 _]
        tunnel: w499 -> [w509 _]
        tunnel: w498 -> [w517 _]
        tunnel: [w506 w521] -> w492
        tunnel: [w513 w520] -> w494
        tunnel: [w507 w519] -> w490
        tunnel: w488 -> [w505 w519]
        frame No Error {
          n153 = call "AlliGator Settings Storage.vi"("AlliGator Settings List"=AlliGator_Settings_List."Data Information:Background Scaling Factor") -> ("Error Out"=w511:errorcluster, "Variant Data out"=w515:variant)  [unwired: 9 in]
          n154 = call-poly "Variant to Data.vi"("Variant"=w515) -> ("Value"=w508:dbl)  [unwired: 8 in]
          n155 = call "AlliGator Subtract Background Image(s) v4.vi"("error in (no error)"=w511, "Background Gate Images, Min, Max & Sum 2"=w509, "Background Gate Images, Min, Max & Sum 1"=w510, "AlliGator IV DVR in"=w512) -> ("error out"=w514:errorcluster, "AlliGator IV DVR out"=w513:refnum<data-value>)  [unwired: 6 in]
          n156 = Format Into String(format string="\nSubtracted background file: %s\nScaling Factor: %#g", initial string=w505, error in=w514, w517, w508) -> (resulting string=w507:string, error out=w506:errorcluster)
        }
        frame Error {
        }
      }
      n157 = call "Hide Animated Busy Icon with Message and Abort Button.vi"("Already active? (F)"=w489, "Target VI reference"=w496, "Error In"=w492) -> ("Error Out"=w497:errorcluster)  [unwired: 16 in]
    }
  }
  "error out" <- w1
  "Script out" <- w15
  "AlliGator Q Elements out" <- w14
  "AlliGator IV DVR" <- w9
  n158 = call "Get Current Message Text Format.vi"("Text Format"=Text_Format_List."Message") -> ("Error Out"=w2:errorcluster, "Message Formatting"=w5:T3)  [unwired: 8 in]
  n159 = call "AlliGator Package Notebook Messages.vi"("Error In"=w2, "Message Formatting"=w5, "Message"=w6, "AlliGator Q Event in"="AlliGator Q Event in") -> ("[Notebook Message]"=→"[Notebook Message]":T2[])  [unwired: 6 in, 1 out]
